vi "winchcontrol2014_TTide_Altimeter_Improved_20150213.vi"() -> ()   [LabVIEW 2014]
uses:
  Instance           1 20Saved   winchcontrol .vi
  Instance           2 20Saved   winchcontrol .vi
  Instance           4 20Saved   winchcontrol .vi
  Instance           3 20Saved   winchcontrol .vi
  isPlaying.vi
  Instance           5 20Saved   winchcontrol .vi
  Instance           6 20Saved   winchcontrol .vi
panel:
  in  "Going up? \ntry to stop at current depth":bool
  out "Too late":string="Too late now!!!  Just pray!"
  out "Current Range":dbl
  out "Fake altimeter yaxis":T1(graph)
  in  "Auto\ndrop":bool
  in  "Final out speed\n[turns/sec]":dbl=4.0 min=0.0 max=4.0 step=0.1 format="%.1f"
  out "pressure":dbl
  out "Dz/Dt":T1(graph)
  out "Payout History":T1(graph)
  out "Conductivity":T1(graph)
  out "Alti Range":T1(graph)
  in  "Path of Image Capture":path=path "/OPG_Winch_MiniCoreDuo/Users/opg/Sites/FCTD_WINCH/LabView.png"
  in  "Screen Capture":bool
  out "Last update string":string="Updated: 10/29/12 6:37:41 PM"
  in  "Port":i32=4050
  in  "Red Lion IP Address":string="192.168.1.160"
  in  "Beep\non wait?":bool=TRUE
  in  "Drive by \nCTD Data":bool=TRUE
  in  "Max. depth [m]":dbl=330.0 min=0.0 max=2200.0 step=1.0 format="%#_4f"
  out "Time @ max":timestamp=timestamp(3434357554.995505 s since 1904-01-01) format="%<%H:%M:%S>T"
  out "Max payout":dbl=26.1 format="%#4.0f"
  out "Max depth":dbl format="%#4.0f"
  in  "Go Up Now":bool
  in  "Final in speed\n[turns/sec]":dbl=0.7 min=0.0 max=4.0 step=0.1 format="%_2f"
  in  "Slow payout (up)\n[turns]":dbl=7.0 min=0.0 max=1500.0 step=1.0
  out "Final in speed":dbl=0.7 min=0.0 max=4.0 step=0.1 format="%3_2g"
  out "Slow payout (up)":dbl=7.0 min=0.0 max=4.0 step=0.1
  out "CTD Miss Count":dbl
  out "Winch Miss Count":dbl=1.0
  out "Sax Status":u8[](array[numeric])=[1, 1, 0, 0, 5, 0, 1, 1, 0, 0]
  out "Depth":T1(graph)
  out "i value":i32
  out "Concat. string":string="$OPGST,1,2,1243"
  out "CTD data":string="2615984408,1.818078,23.842880,5.097004"
  out "Depth":dbl(slide)=1.8080824462346528 min=0.0 max=1200.0 scale format="%#_4f"
  out "*(type *) &x":i32=38
  out "timestamp":u32=2615984408
  out "Temperature":T1(graph)
  out "Param. String":string="$reqparmx:0019;0000$OPGWPM,10,16,+   6,+ 500, 4.2, 2.0,10000,10000,20000,40000,60000,60000,    0.70,    7,;"
  out "Status String":string="$OPGWST,3,1,+   1.8, 266.9,   0,- 0.01,   0.00,   0,   26307,;"
  out "Sax Status Code":dbl=26307.0 format="%#_8f"
  out "Motor Current":dbl
  out "Motor Payout":dbl=266.9
  out "Sheave Payout":dbl
  out "ATM90 Payout":dbl=1.8
  in  "CTD Data  IP Address":string="192.168.1.158"
  in  "Port":i32=2342
  out "bytes written":i32=62
  out "RL Status Received":bool=TRUE
  out "Accel out":dbl=10000.0
  out "Accel in":dbl=10000.0
  out "Winch Action Status":T2(ring)=enum."HOMING"
  out "Winch Control Mode":u16(ring)=3 items=["STOPPED", "MANUAL JOY", "MANUAL POT", "AUTO", "SEMIAUTO"]
  out "Decel stop in":dbl=60000.0
  out "Decel stop out":dbl=60000.0
  out "Decel in":dbl=40000.0
  out "Decel out":dbl=20000.0
  out "Wire in speed":dbl=2.0
  out "Wire out speed":dbl=4.2
  out "Min payout":dbl=6.0
  out "Max payout":dbl=500.0
  out "Current limit out":dbl=10.0
  out "Current limit in":dbl=16.0
  in  "Drop time [min.]":dbl=8.099999999999985 min=0.0 step=0.1 format="%.1f"
  out "output":string
  in  "Stop Now":bool
  in  "Wire in speed\n[turns/sec]":dbl=2.0 min=0.0 max=5.0 step=0.1 format="%3_2f"
  in  "Decel in":dbl=40000.0
  in  "Decel out":dbl=20000.0
  in  "Stop decel in":dbl=60000.0
  in  "Stop decel out":dbl=60000.0
  in  "Accel  in":dbl=10000.0
  in  "Accel out":dbl=10000.0
  in  "Current limit out\n[Amps]":dbl=10.0 min=0.0 max=20.0 step=0.1 format="%_3f"
  in  "Current limit in\n[Amps]":dbl=16.0 min=0.0 max=19.5 format="%_3f"
  out "input":string="$reqparmx:0019;0000$OPGWPM,10,16,+   6,+ 500, 4.2, 2.0,10000,10000,20000,40000,60000,60000,    0.70,    7,;"
  out "Payout":dbl(slide)=1.8 min=0.0 max=1200.0 step=200.0 scale format="%#1_3f"
  out "Velocity Now":dbl(knob)=-0.01 min=-5.0 max=5.0 step=1.0 scale=-5.0..5.0 scale format="%#_1f"
  in  "Max. payout [turns]":dbl=500.0 min=0.0 max=1640.0 step=1.0 format="%#_4f"
  in  "Min. payout [turns]":dbl=6.0 min=0.0 max=2000.0 step=1.0
  in  "Winch Auto Run":bool=TRUE
  out "Enabled":bool=TRUE
  in  "Vel out Init. [turns/sec]":dbl=4.2 min=0.0 max=8.0 step=0.1 format="%_2f"
  out "Target\nDepth":dbl
  # "OPG  FastCTD LabVIEW CONTROLLER"
  # "Winch Variable Controls"
  # "Winch Variable Status"
  # "Communication Setup"
  # "Communication Data"
  # "FCTD DATA"
  # "RED LION CONTROL"
  # "Screen Capture"
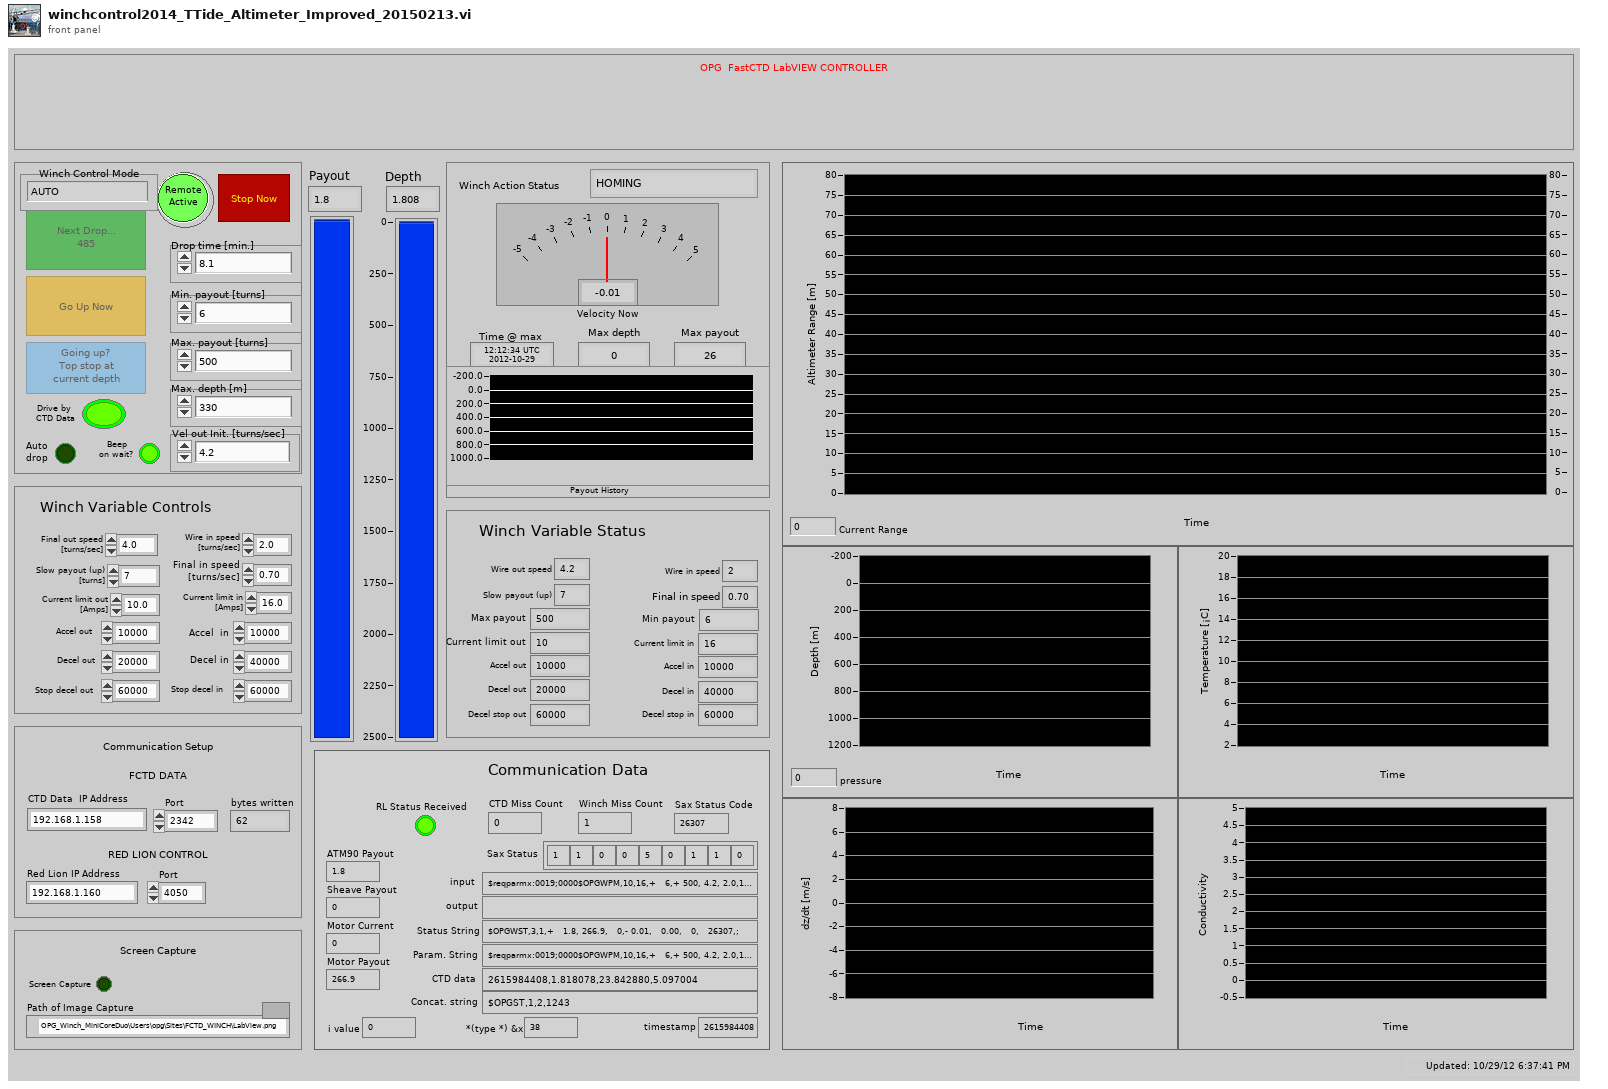
[diagram p1: front panel]
types:
  T1 = cluster{"seconds since 1Jan1904":timestamp, dbl}[]
  T2 = enum16{"START HOMING", "HOMING", "WAIT FOR TRIGGER", "START DROP", "GOING DOWN ?", "GOING UP"}
  T3 = cluster{"Array[0]":dbl, "Array[1]":dbl, "Array[2]":dbl, "Array[3]":dbl, "Array[4]":dbl, "Array[5]":dbl, "Array[6]":dbl, "Array[7]":dbl, "Array[8]":dbl}
  T4 = cluster{"Array[0]":dbl, "Array[1]":dbl, "Array[2]":dbl, "Array[3]":dbl, "Array[4]":dbl, "Array[5]":dbl, "Array[6]":dbl, "Array[7]":dbl, "Array[8]":dbl, "Array[9]":dbl, "Array[10]":dbl, "Array[11]":dbl, "Array[12]":dbl, "Array[13]":dbl}
  T5 = typedef "imagedata.ctl" = cluster{"image type":i32, "image depth":i32, "image":u8[], "mask":u8[], "colors":u32[], "Rectangle":cluster{"left":i16, "top":i16, "right":i16, "bottom":i16}}
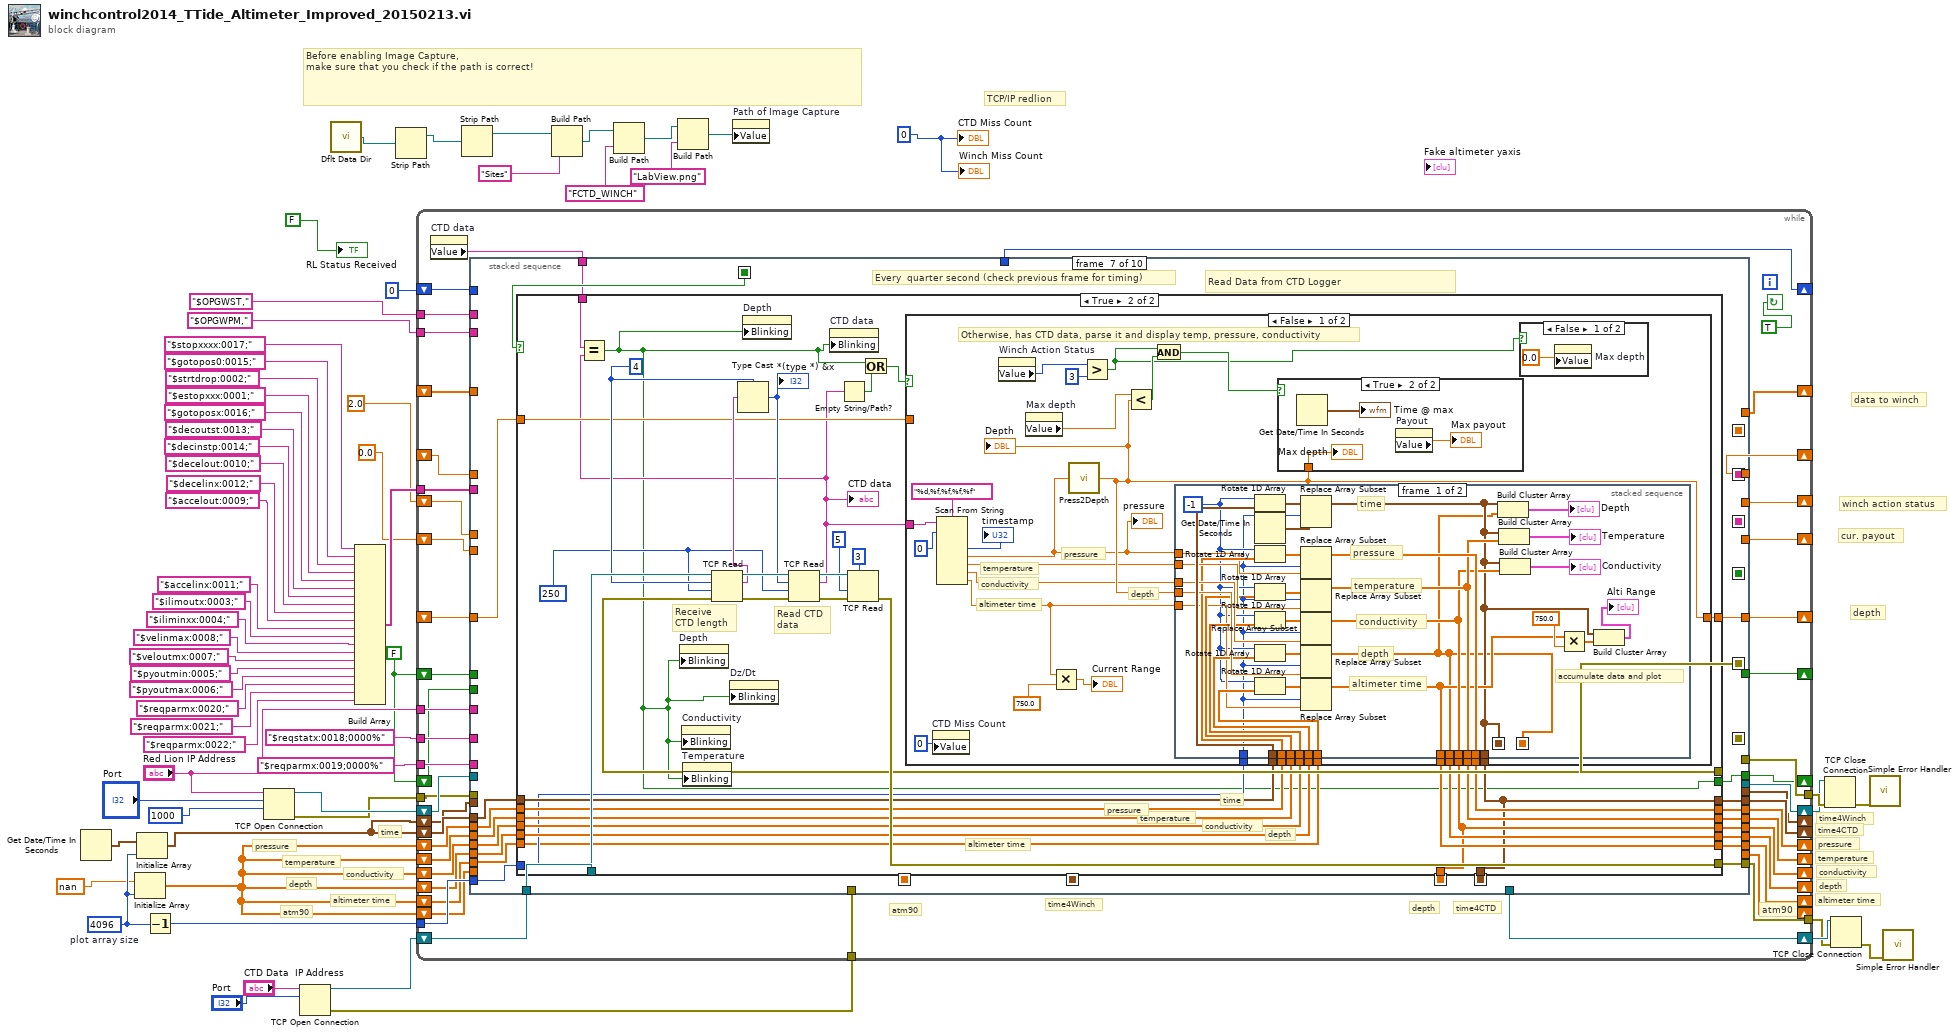
[diagram p0: block diagram]
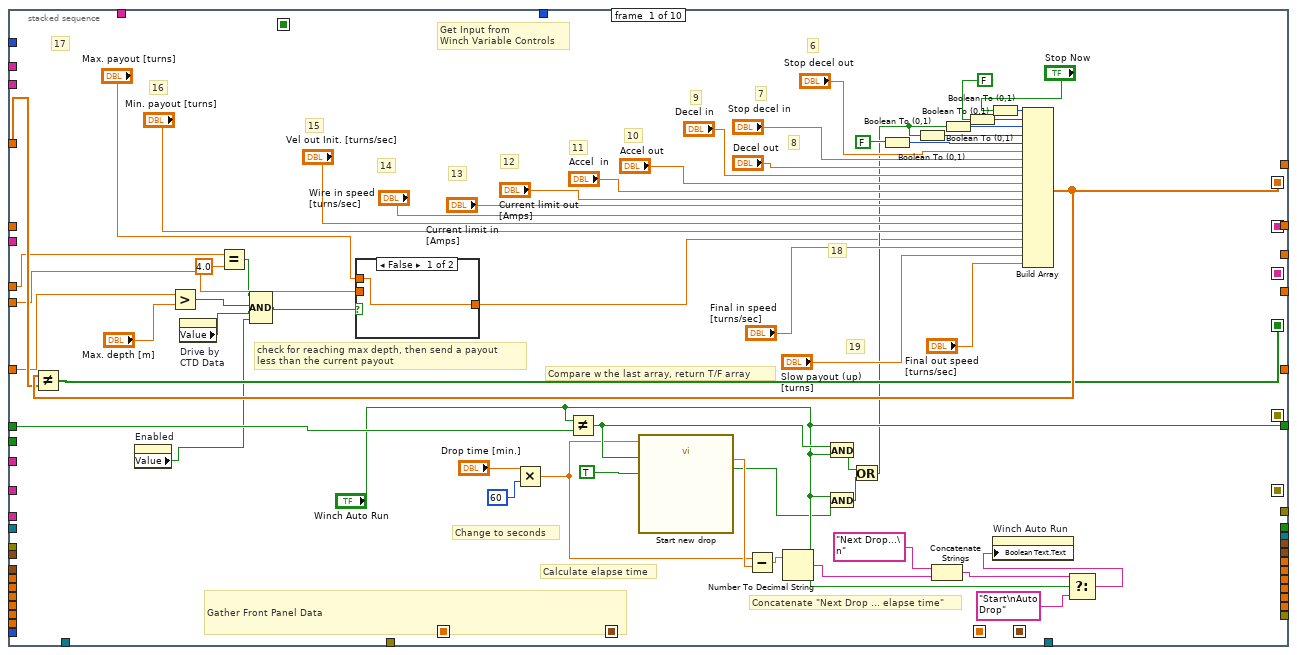
[diagram p2: hidden frame]
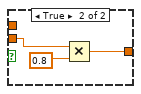
[diagram p3: hidden frame]
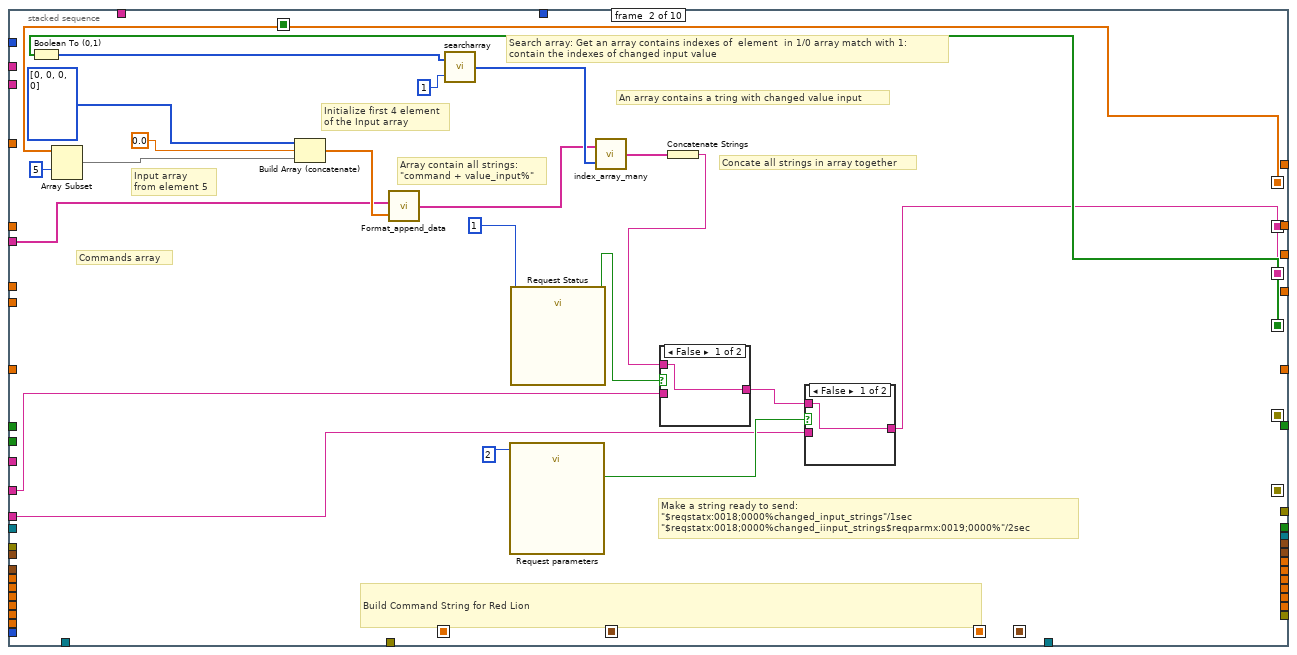
[diagram p4: hidden frame]
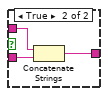
[diagram p5: hidden frame]
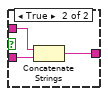
[diagram p6: hidden frame]
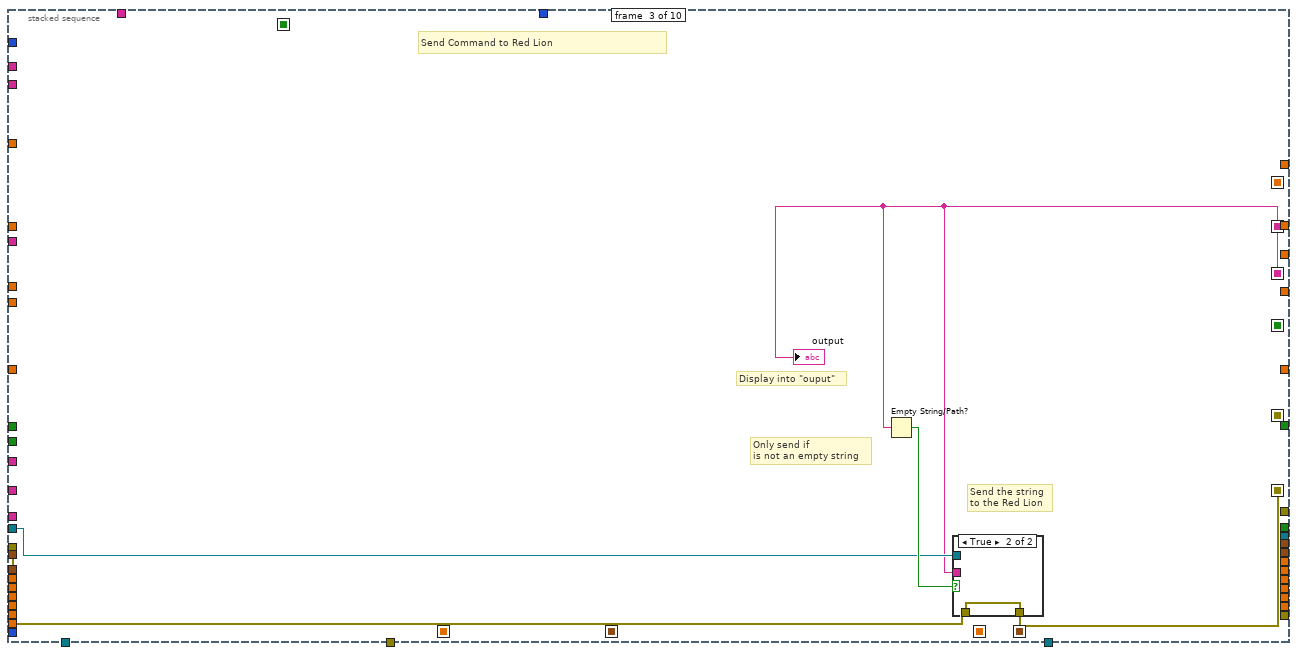
[diagram p7: hidden frame]
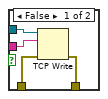
[diagram p8: hidden frame]
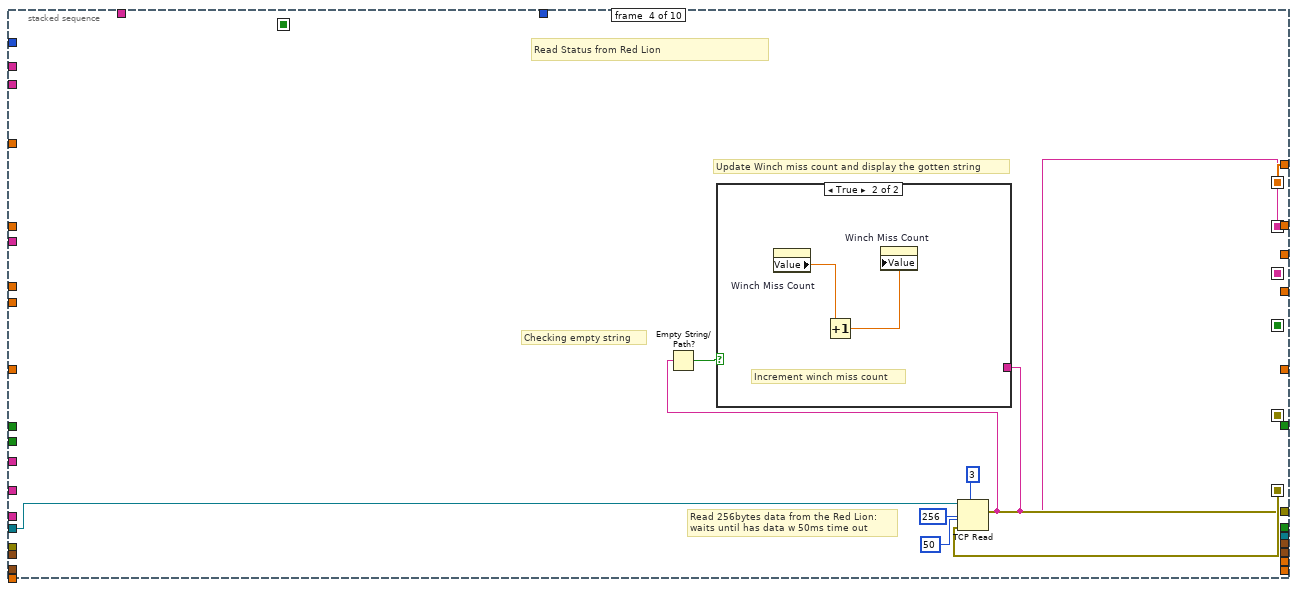
[diagram p9: hidden frame]
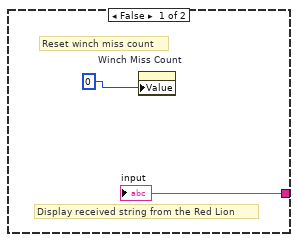
[diagram p10: hidden frame]
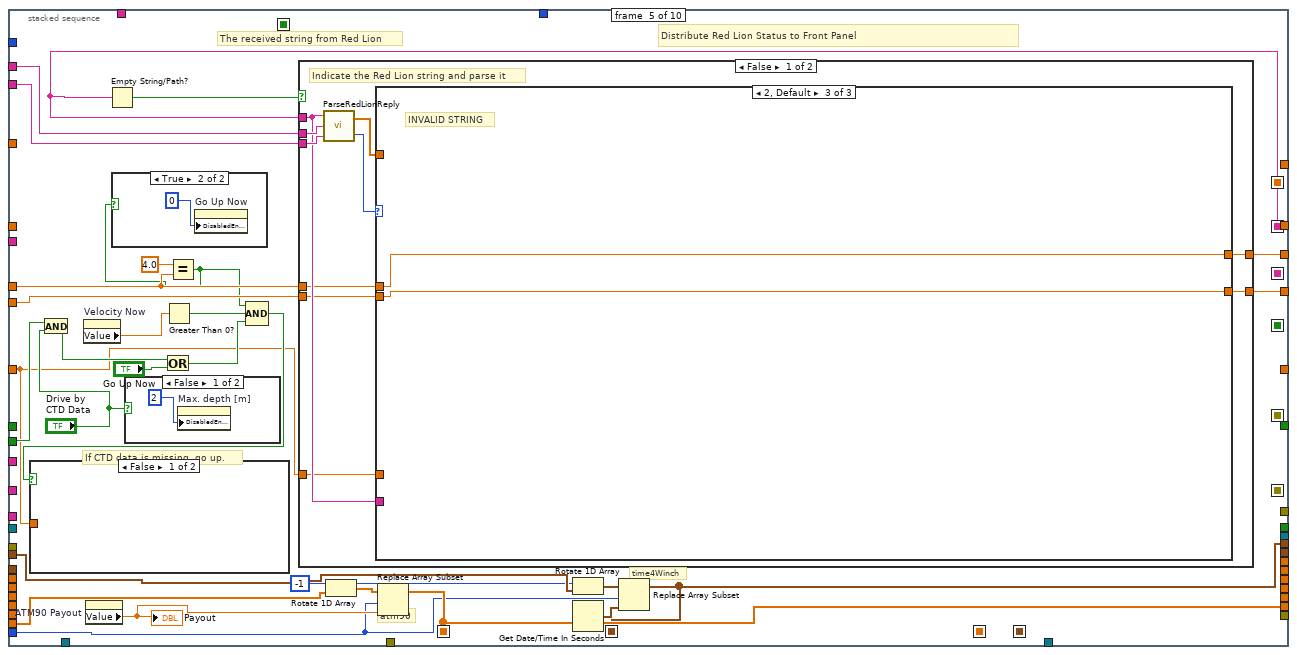
[diagram p11: hidden frame]
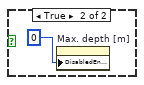
[diagram p12: hidden frame]
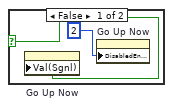
[diagram p13: hidden frame]
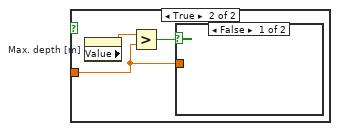
[diagram p14: hidden frame]
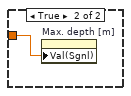
[diagram p15: hidden frame]
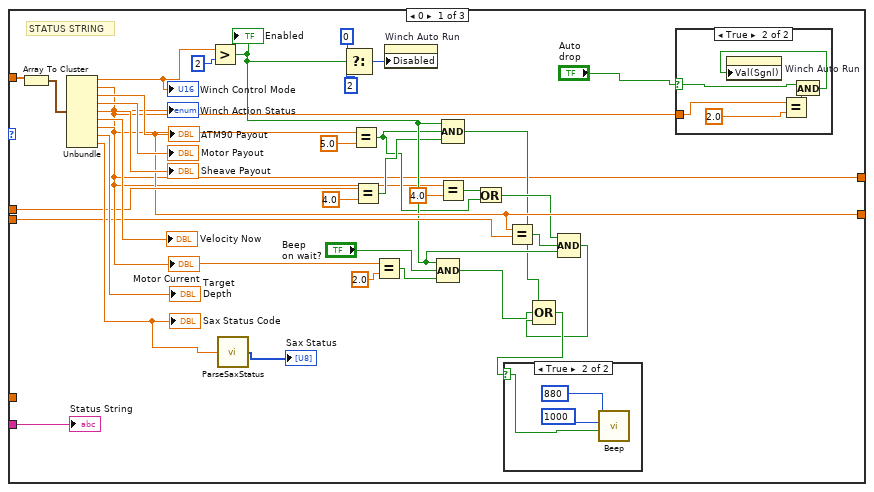
[diagram p16: hidden frame]
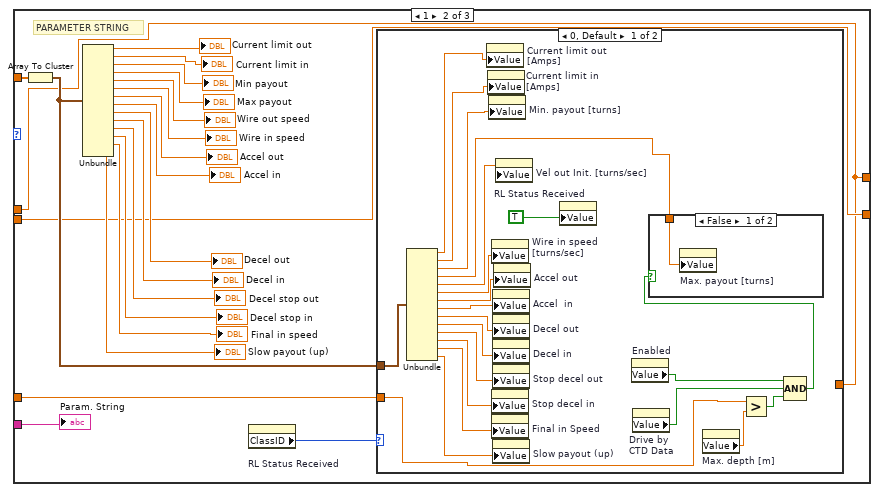
[diagram p19: hidden frame]
diagram:
  w6 = 4096  # plot array size
  w19 = FALSE
  w25 = 0
  # "cur. payout"
  # "depth"
  # "data to winch"
  # "winch action status"
  # "time4Winch"
  # "atm90"
  # "depth"
  # "altimeter time"
  # "altimeter time"
  # "conductivity"
  # "temperature"
  # "time4CTD"
  # "pressure"
  # "depth"
  # "conductivity"
  # "temperature"
  # "time"
  # "pressure"
  # "Before enabling Image Capture, \nmake sure that you check if the path is correct!"
  # "TCP/IP redlion"
  n1 = Get Date/Time In Seconds() -> (seconds since 1Jan1904=w5:timestamp)
  n2 = Initialize Array(nan, w6) -> (w4:dbl[])
  n3 = Initialize Array(w5, w6) -> (w3:timestamp[])
  n4 = Decrement(x=w6) -> (x-1=w7:i32)
  n5 = TCP Open Connection(address="Red Lion IP Address", remote port or service name="Port", timeout ms (60000)=1000) -> (connection ID=w60:refnum<k5>, error out=w58:errorcluster)  [unwired: 2 in]
  n6 = TCP Open Connection(address="CTD Data  IP Address", remote port or service name="Port") -> (connection ID=w34:refnum<k5>, error out=w32:errorcluster)  [unwired: 3 in]
  n7 = call <vilib>:"Dflt Data Dir.vi"() -> ("App:Default Data Directory"=w16:path)
  n8 = Build Array("$stopxxxx:0017;", "$gotopos0:0015;", "$strtdrop:0002;", "$estopxxx:0001;", "$gotoposx:0016;", "$decoutst:0013;", "$decinstp:0014;", "$decelout:0010;", "$decelinx:0012;", "$accelout:0009;", "$accelinx:0011;", "$ilimoutx:0003;", "$iliminxx:0004;", "$velinmax:0008;", "$veloutmx:0007;", "$pyoutmin:0005;", "$pyoutmax:0006;", "$reqparmx:0020;", "$reqparmx:0021;", "$reqparmx:0022;") -> (w56:string[])
  n9 = Strip Path(path=w16) -> (stripped path=w15:path)  [unwired: 1 out]
  n10 = while {
    shift-right: [w110] -> _
    shift-left: _ -> [w108]
    tunnel: w58 -> [w105]
    tunnel: [w109] -> w57
    tunnel: w56 -> [w107]
    tunnel: "$reqstatx:0018;0000%" -> [w104]
    shift-right: [w103] -> _
    shift-left: w19 -> [w102]
    tunnel: w32 -> [w100]
    tunnel: [w99] -> w31
    tunnel: "$reqparmx:0019;0000%" -> [w98]
    shift-right: [w97] -> _
    shift-left: _ -> [w96]
    shift-right: [w95] -> _
    shift-left: 0 -> [w94]
    tunnel: "$OPGWST," -> [w93]
    tunnel: "$OPGWPM," -> [w92]
    shift-right: [w90] -> w24
    shift-left: w60 -> [w106]
    shift-right: [w89] -> w33
    shift-left: w34 -> [w101]
    shift-right: [w88] -> _
    shift-left: _ -> [w87]
    tunnel: "Red Lion IP Address" -> [w85]
    shift-right: [w84] -> _
    shift-left: w19 -> [w83]
    shift-right: [w82] -> _
    shift-left: 2.0 -> [w81]
    shift-right: [w80] -> _
    shift-left: 0.0 -> [w79]
    tunnel: w7 -> [w78]
    shift-right: [w70] -> _
    shift-left: w4 -> [w76]
    shift-right: [w72] -> _
    shift-left: w3 -> [w77]
    shift-right: [w69] -> _
    shift-left: w4 -> [w75]
    shift-right: [w67] -> _
    shift-left: w4 -> [w74]
    shift-right: [w68] -> _
    shift-left: w4 -> [w73]
    shift-right: [w66] -> _
    shift-left: w4 -> [w71]
    shift-right: [w64] -> _
    shift-left: w4 -> [w65]
    shift-right: [w62] -> _
    shift-left: w3 -> [w63]
    stop <- TRUE continue-if-true
    # "time4CTD"
    # "time4Winch"
    # "depth"
    # "atm90"
    # "atm90"
    n11 = property on="CTD data" class="Str"() -> ("Value"=w86:string)  [unwired: 2 in, 2 out]
    n12 = stacked-sequence {
      seq-local: [w165 _ _ _ _ _ _ _ _ _] -> [_ w184 _ w218 _ _ _ _ _ _]
      seq-local: [_ w170 _ _ _ _ _ _ _ _] -> [_ _ w200 _ _ _ _ _ _ _]
      seq-local: [_ _ w201 _ _ _ _ _ _ _] -> [_ _ _ w213 _ _ _ _ _ _]
      seq-local: [w161 _ _ _ _ _ _ _ _ _] -> [_ w191 _ _ _ _ _ _ _ _]
      seq-local: [_ _ _ w211 _ _ _ _ _ _] -> [_ _ _ _ w249 _ _ _ _ _]
      seq-local: [_ _ _ _ _ w369 _ _ _ _] -> [_ _ _ _ _ _ w429 _ _ _]
      seq-local: [_ _ _ _ _ w368 _ _ _ _] -> [_ _ _ _ _ _ w427 _ _ _]
      seq-local: [_ _ _ _ _ _ w409 _ _ _] -> [_ _ _ _ _ _ _ _ _ w662]
      seq-local: [_ _ _ _ w233 _ _ _ _ _] -> [_ _ _ _ _ _ _ _ _ w663]
      seq-local: [_ _ _ _ w228 _ _ _ _ _] -> [_ _ _ _ _ _ _ _ _ w661]
      seq-local: [_ _ _ _ _ _ w408 _ _ _] -> [_ _ _ _ _ _ _ _ _ w660]
      tunnel: w105 -> [_ _ w203 _ _ _ _ _ _ _]
      tunnel: w106 -> [_ _ w202 w214 _ _ _ _ w625 _]
      tunnel: [_ _ _ w218 _ _ _ _ _ _] -> w110
      tunnel: w107 -> [_ w182 _ _ _ _ _ _ _ _]
      tunnel: [_ _ _ w212 _ _ _ _ _ _] -> w109
      tunnel: w108 -> [w164 _ _ _ _ _ _ _ _ _]
      tunnel: w104 -> [_ w176 _ _ _ _ _ _ _ _]
      tunnel: ["Winch Auto Run" _ _ _ _ _ _ _ _ _] -> w103
      tunnel: w102 -> [w141 _ _ _ _ _ _ _ _ _]
      tunnel: w101 -> [_ _ _ _ _ w371 w430 _ w623 _]
      tunnel: w100 -> [_ _ _ _ _ w370 _ _ _ _]
      tunnel: [_ _ _ _ _ _ w428 _ _ _] -> w99
      tunnel: w98 -> [_ w171 _ _ _ _ _ _ _ _]
      tunnel: [_ _ _ _ _ w367 _ _ _ _] -> w97
      tunnel: w96 -> [_ _ _ _ _ w366 _ _ _ _]
      tunnel: w94 -> [_ _ _ _ _ w365 _ _ _ _]
      tunnel: [_ _ _ _ _ w364 _ _ _ _] -> w95
      tunnel: w93 -> [_ _ _ _ w251 _ _ _ _ _]
      tunnel: w92 -> [_ _ _ _ w250 _ _ _ _ _]
      tunnel: [_ _ _ _ _ _ _ _ w624 _] -> w90
      tunnel: [_ _ _ _ _ _ _ _ w622 _] -> w89
      tunnel: [_ _ _ _ _ _ w426 _ _ _] -> w88
      tunnel: w87 -> [w121 _ _ _ w223 _ w425 _ _ _]
      tunnel: w86 -> [_ _ _ _ _ _ w424 _ _ _]
      tunnel: w85 -> [_ _ _ _ _ _ _ _ w621 _]
      tunnel: [_ _ _ _ _ _ w423 _ _ _] -> w84
      tunnel: w83 -> [_ _ _ _ w227 _ _ _ _ _]
      tunnel: [_ _ _ _ w243 _ _ _ _ _] -> w82
      tunnel: w81 -> [w112 _ _ _ w239 _ _ _ _ _]
      tunnel: [_ _ _ _ w242 _ _ _ _ _] -> w80
      tunnel: w79 -> [w118 _ _ _ w241 _ _ _ _ _]
      tunnel: w78 -> [_ _ _ _ w230 _ w422 _ _ _]
      tunnel: w77 -> [_ _ _ _ _ _ w421 _ _ _]
      tunnel: w76 -> [_ _ _ _ _ _ w420 _ _ _]
      tunnel: w75 -> [_ _ _ _ _ _ w419 _ _ _]
      tunnel: w74 -> [_ _ _ _ _ _ w418 _ _ _]
      tunnel: w73 -> [_ _ _ _ _ _ w417 _ _ _]
      tunnel: [_ _ _ _ _ _ w416 _ _ _] -> w72
      tunnel: w71 -> [_ _ _ _ _ _ w415 _ _ _]
      tunnel: [_ _ _ _ _ _ w414 _ _ _] -> w70
      tunnel: [_ _ _ _ _ _ w413 _ _ _] -> w69
      tunnel: [_ _ _ _ _ _ w412 _ _ _] -> w67
      tunnel: [_ _ _ _ _ _ w411 _ _ _] -> w68
      tunnel: [_ _ _ _ _ _ w410 _ _ _] -> w66
      tunnel: w65 -> [_ _ _ _ w237 _ _ _ _ _]
      tunnel: [_ _ _ _ w233 _ _ _ _ _] -> w64
      tunnel: w63 -> [_ _ _ _ w232 _ _ _ _ _]
      tunnel: [_ _ _ _ w228 _ _ _ _ _] -> w62
      frame #0 {
        w162 = FALSE items=["OFF", "ON", "OFF", "ON"] ("Return to top")
        w150 = FALSE items=["OFF", "ON", "OFF", "ON"] ("Go to ...")
        # "check for reaching max depth, then send a payout\nless than the current payout"
        # "19"
        # "18"
        # "17"
        # "16"
        # "15"
        # "14"
        # "13"
        # "12"
        # "11"
        # "10"
        # "9"
        # "8"
        # "7"
        # "6"
        # "Compare w the last array, return T/F array"
        # "Concatenate \"Next Drop ... elapse time\""
        # "Calculate elapse time"
        # "Change to seconds"
        # "Get Input from\nWinch Variable Controls"
        # "Gather Front Panel Data"
        n13 = property on="Enabled" class="Bool (strict)"() -> ("Value"=w115:bool)  [unwired: 2 in, 2 out]
        n14 = Greater?(x=w121, y="Max. depth [m]") -> (0:w117:bool)
        n15 = property on="Drive by \nCTD Data" class="Bool (strict)"() -> ("Value"=w116:bool)  [unwired: 2 in, 2 out]
        n16 = Equal?(x=w112, y=4.0) -> (x = y?=w111:bool)
        n17 = Compound Arithmetic op=AND(w111, w117, w116, w115) -> (w114:bool)
        n18 = case shown="False" w114 {
          tunnel: "Max. payout [turns]" -> [w166 _]
          tunnel: [w166 w168] -> w119
          tunnel: w118 -> [_ w167]
          frame False {
          }
          frame True {
            n19 = Multiply(x=w167, y=0.8) -> (x*y=w168:dbl)
          }
        }
        n20 = Multiply(x="Drop time [min.]", y=60) -> (x*y=w136:dbl)
        n21 = Not Equal?(x="Winch Auto Run", y=w141) -> (x != y?=w140:bool)
        n22 = call "Start new drop"("Time Target (s)"=w136, "Reset"=w140, "Auto Reset"=TRUE) -> ("Elapsed Time (s)"=w137:dbl, "Time has Elapsed"=w126:bool)  [unwired: 9 in, 6 out]
        n23 = Subtract(x=w136, y=w137) -> (x-y=w135:dbl)
        n24 = Number To Decimal String(number=w135) -> (decimal integer string=w134:string)  [unwired: 1 in]
        n25 = And(x=w140, y="Winch Auto Run") -> (x .and. y?=w139:bool)
        n26 = And(x="Winch Auto Run", y=w126) -> (x .and. y?=w138:bool)
        n27 = Or(x=w139, y=w138) -> (x .or. y?=w124:bool)
        n28 = Boolean To (0,1)(Boolean=w150) -> (0, 1=w149:i16)
        n29 = Boolean To (0,1)(Boolean=w124) -> (0, 1=w148:i16)
        n30 = Concatenate Strings("Next Drop...\n", w134) -> (w131:string)
        n31 = Boolean To (0,1)(Boolean=w124) -> (0, 1=w147:i16)
        n32 = Boolean To (0,1)(Boolean=w162) -> (0, 1=w146:i16)
        n33 = Boolean To (0,1)(Boolean="Stop Now") -> (0, 1=w145:i16)
        n34 = Build Array(w145, w146, w147, w148, w149, "Stop decel out", "Stop decel in", "Decel out", "Decel in", "Accel out", "Accel  in", "Current limit out\n[Amps]", "Current limit in\n[Amps]", "Wire in speed\n[turns/sec]", "Vel out Init. [turns/sec]", "Min. payout [turns]", w119, "Final in speed\n[turns/sec]", "Slow payout (up)\n[turns]", "Final out speed\n[turns/sec]") -> (w165:dbl[])
        n35 = Not Equal?(x=w165, y=w164) -> (x != y?=w161:bool[])
        n36 = Select(t=w131, s="Winch Auto Run", f="Start\nAuto Drop") -> (s? t:f=w132:string)
        n37 = property on="Winch Auto Run" class="Bool (strict)"("Boolean Text.Text"=w132) -> ()  [unwired: 2 in, 2 out]
      }
      frame #1 {
        # "Make a string ready to send:\n\"$reqstatx:0018;0000%changed_input_strings\"/1sec\n\"$reqstatx:0018;0000%changed_iinput_strings$reqparmx:0019;0000%\"/2sec"
        # "Concate all strings in array together"
        # "An array contains a tring with changed value input"
        # "Array contain all strings:\n\"command + value_input%\""
        # "Commands array"
        # "Initialize first 4 element\nof the Input array"
        # "Input array\nfrom element 5"
        # "Search array: Get an array contains indexes of  element  in 1/0 array match with 1:\ncontain the indexes of changed input value"
        # "Build Command String for Red Lion"
        n38 = Boolean To (0,1)(Boolean=w191) -> (0, 1=w189:i16[])
        n39 = Array Subset(array=w184, index=5) -> (w180:dbl[])  [unwired: 1 in]
        n40 = Build Array (concatenate)(i32[] [0, 0, 0, 0], 0.0 ("Depth to go to"), w180) -> (w183:dbl[])
        n41 = call "Format_append_data.vi"("Numbers to append"=w183, "Strings without numbers"=w182) -> ("Final Strings"=w181:string[])
        n42 = call "searcharray.vi"("Search character"=1, "Array 2"=w189) -> ("Array"=w188:i16[])
        n43 = call "Request parameters"("Time Target (s)"=2) -> ("Time has Elapsed"=w172:bool)  [unwired: 11 in, 7 out]
        n44 = call "Request Status"("Time Target (s)"=1) -> ("Time has Elapsed"=w177:bool)  [unwired: 11 in, 7 out]
        n45 = call "index_array_many.vi"("Lines of Array to grab"=w188, "String Array Input"=w181) -> ("Output array"=w187:string[])
        n46 = Concatenate Strings(w187) -> (w175:string)
        n47 = case shown="False" w177 {
          tunnel: w175 -> [w196 w199]
          tunnel: [w196 w198] -> w173
          tunnel: w176 -> [_ w197]
          frame False {
          }
          frame True {
            n48 = Concatenate Strings(w199, w197) -> (w198:string)
          }
        }
        n49 = case shown="False" w172 {
          tunnel: w173 -> [w192 w195]
          tunnel: [w192 w194] -> w170
          tunnel: w171 -> [_ w193]
          frame False {
          }
          frame True {
            n50 = Concatenate Strings(w195, w193) -> (w194:string)
          }
        }
      }
      frame #2 {
        # "Send the string\nto the Red Lion"
        # "Only send if\nis not an empty string"
        # "Display into \"ouput\""
        # "Send Command to Red Lion"
        n51 = Empty String/Path?(string/path=w200) -> (empty?=w204:bool)
        n52 = case shown="True" w204 {
          tunnel: w200 -> [w207 _]
          tunnel: w202 -> [w208 _]
          tunnel: w203 -> [w206 w209]
          tunnel: [w205 w209] -> w201
          frame False {
            n53 = TCP Write(connection ID=w208, data in=w207, error in (no error)=w206) -> (error out=w205:errorcluster)  [unwired: 1 in, 2 out]
          }
          frame True {
          }
        }
        "output" <- w200
      }
      frame #3 {
        # "Update Winch miss count and display the gotten string"
        # "Checking empty string"
        # "Read 256bytes data from the Red Lion:\nwaits until has data w 50ms time out"
        # "Read Status from Red Lion"
        n54 = TCP Read(connection ID=w214, bytes to read=256, error in (no error)=w213, 7:3, 9:50) -> (data out=w211:string, error out=w212:errorcluster)  [unwired: 1 out]
        n55 = Empty String/Path?(string/path=w211) -> (empty?=w210:bool)
        n56 = case shown="True" w210 {
          tunnel: w211 -> [w220 _]
          frame False {
            # "Display received string from the Red Lion"
            # "Reset winch miss count"
            n57 = property on="Winch Miss Count" class="DigNum (strict)"("Value"=0) -> ()  [unwired: 2 in, 2 out]
            "input" <- w220
          }
          frame True {
            # "Increment winch miss count"
            n58 = property on="Winch Miss Count" class="DigNum (strict)"() -> ("Value"=w222:dbl)  [unwired: 2 in, 2 out]
            n59 = Increment(x=w222) -> (x+1=w221:dbl)
            n60 = property on="Winch Miss Count" class="DigNum (strict)"("Value"=w221) -> ()  [unwired: 2 in, 2 out]
          }
        }
      }
      frame #4 {
        w231 = -1
        # "If CTD data is missing, go up."
        # "time4Winch"
        # "atm90"
        # "The received string from Red Lion"
        # "Distribute Red Lion Status to Front Panel"
        n61 = And(x=w227, y="Drive by \nCTD Data") -> (x .and. y?=w226:bool)
        n62 = property on="Velocity Now" class="Knob (strict)"() -> ("Value"=w247:dbl)  [unwired: 2 in, 2 out]
        n63 = property on="ATM90 Payout" class="DigNum (strict)"() -> ("Value"=w235:dbl)  [unwired: 2 in, 2 out]
        "Payout" <- w235
        n64 = Empty String/Path?(string/path=w249) -> (empty?=w248:bool)
        n65 = case shown="False" "Drive by \nCTD Data" {
          frame False {
            n66 = property on="Max. depth [m]" class="DigNum (strict)"("DisabledEnum"=2) -> ()  [unwired: 2 in, 2 out]
          }
          frame True {
            n67 = property on="Max. depth [m]" class="DigNum (strict)"("DisabledEnum"=0) -> ()  [unwired: 2 in, 2 out]
          }
        }
        n68 = Or(x=w226, y="Go Up Now") -> (x .or. y?=w244:bool)
        n69 = Greater Than 0?(x=w247) -> (x > 0?=w245:bool)
        n70 = Equal?(x=4.0, y=w239) -> (x = y?=w238:bool)
        n71 = case shown="True" w238 {
          selector: w238 -> [w254 _]
          frame False {
            n72 = property on="Go Up Now" class="Bool (strict)"("Val(Sgnl)"=w254) -> ()  [unwired: 2 in, 2 out]
            n73 = property on="Go Up Now" class="Bool (strict)"("DisabledEnum"=2) -> ()  [unwired: 2 in, 2 out]
          }
          frame True {
            n74 = property on="Go Up Now" class="Bool (strict)"("DisabledEnum"=0) -> ()  [unwired: 2 in, 2 out]
          }
        }
        n75 = Compound Arithmetic op=AND(w238, w245, w244) -> (w246:bool)
        n76 = case shown="False" w246 {
          tunnel: w223 -> [_ w257]
          frame False {
          }
          frame True {
            n77 = property on="Max. depth [m]" class="DigNum (strict)"() -> ("Value"=w259:dbl)  [unwired: 2 in, 2 out]
            n78 = Greater?(x=w259, y=w257) -> (0:w258:bool)
            n79 = case shown="False" w258 {
              tunnel: w257 -> [_ w260]
              frame False {
              }
              frame True {
                n80 = property on="Max. depth [m]" class="DigNum (strict)"("Val(Sgnl)"=w260) -> ()  [unwired: 2 in, 2 out]
              }
            }
          }
        }
        n81 = case shown="False" w248 {
          tunnel: w251 -> [w268 _]
          tunnel: w250 -> [w267 _]
          tunnel: w249 -> [w266 _]
          tunnel: [w265 w362] -> w243
          tunnel: w239 -> [w264 w362]
          tunnel: [w263 w361] -> w242
          tunnel: w241 -> [w262 w361]
          tunnel: w223 -> [w261 _]
          frame False {
            # "Indicate the Red Lion string and parse it"
            n82 = call "ParseRedLionReply.vi"("Parameter Iidicator"=w267, "Status Indicator"=w268, "Red Lion String"=w266) -> ("Type"=w270:i16, "Array"=w269:dbl[])
            n83 = case shown="2, Default" w270 {
              tunnel: w269 -> [w305 w335 _]
              tunnel: w266 -> [w297 w321 _]
              tunnel: [w272 w316 w360] -> w265
              tunnel: w264 -> [w288 w316 w360]
              tunnel: [w287 w318 w359] -> w263
              tunnel: w262 -> [w286 w318 w359]
              tunnel: w261 -> [_ w315 _]
              frame 0 {
                # "STATUS STRING"
                n84 = Array To Cluster(array=w305) -> (cluster=w304:T3)
                n85 = Unbundle(w304) -> ("Array[0]"=w303:dbl, "Array[1]"=w272:dbl, "Array[2]"=w287:dbl, "Array[3]"=→"Motor Payout":dbl, "Array[4]"=→"Sheave Payout":dbl, "Array[5]"=→"Velocity Now":dbl, "Array[6]"=→"Motor Current":dbl, "Array[7]"=→"Target\nDepth":dbl, "Array[8]"=w293:dbl)
                "Winch Control Mode" <- w303
                "Winch Action Status" <- w272
                "ATM90 Payout" <- w287
                "Sax Status Code" <- w293
                n86 = Greater?(x=w303, y=2) -> (0:w281:bool)
                "Enabled" <- w281
                n87 = call "ParseSaxStatus.vi"("Status Code In"=w293) -> ("Status Flags"=→"Sax Status":i8[])
                n88 = Select(t=0, s=w281, f=2) -> (s? t:f=w294:i32)
                n89 = Equal?(x=w272, y=5.0) -> (x = y?=w274:bool)
                n90 = Equal?(x=w288, y=4.0) -> (x = y?=w278:bool)
                n91 = Equal?(x=w272, y=2.0) -> (x = y?=w280:bool)
                n92 = property on="Winch Auto Run" class="Bool (strict)"("Disabled"=w294) -> ()  [unwired: 2 in, 2 out]
                n93 = Compound Arithmetic op=AND(w281, "Beep\non wait?", w280) -> (w275:bool)
                n94 = Equal?(x=w272, y=4.0) -> (x = y?=w284:bool)
                n95 = Compound Arithmetic op=AND(w281, w274, w278) -> (w277:bool)
                n96 = Or(x=w284, y=w274) -> (x .or. y?=w283:bool)
                n97 = Equal?(x=w287, y=w286) -> (x = y?=w282:bool)
                n98 = Compound Arithmetic op=AND(w283, w282, w281) -> (w273:bool)
                n99 = Compound Arithmetic op=OR(w277, w275, w273) -> (w276:bool)
                n100 = case shown="True" w276 {
                  selector: w276 -> [_ w312]
                  frame False {
                  }
                  frame True {
                    n101 = call <vilib>:"Beep.vi"("use system alert? (T) - ignored"=w312, "duration (msec) - ignored"=u32 1000, "frequency (Hz) - ignored"=u32 880) -> ()  [unwired: 9 in]
                  }
                }
                n102 = case shown="True" "Auto\ndrop" {
                  selector: "Auto\ndrop" -> [_ w308]
                  tunnel: w272 -> [_ w310]
                  frame False {
                  }
                  frame True {
                    n103 = Equal?(x=w310, y=2.0) -> (x = y?=w309:bool)
                    n104 = And(x=w308, y=w309) -> (x .and. y?=w307:bool)
                    n105 = property on="Winch Auto Run" class="Bool (strict)"("Val(Sgnl)"=w307) -> ()  [unwired: 2 in, 2 out]
                  }
                }
                "Status String" <- w297
              }
              frame 1 {
                # "PARAMETER STRING"
                n106 = Array To Cluster(array=w335) -> (cluster=w322:T4)
                n107 = Unbundle(w322) -> ("Array[0]"=→"Current limit out":dbl, "Array[1]"=→"Current limit in":dbl, "Array[2]"=→"Min payout":dbl, "Array[3]"=→"Max payout":dbl, "Array[4]"=→"Wire out speed":dbl, "Array[5]"=→"Wire in speed":dbl, "Array[6]"=→"Accel out":dbl, "Array[7]"=→"Accel in":dbl, "Array[8]"=→"Decel out":dbl, "Array[9]"=→"Decel in":dbl, "Array[10]"=→"Decel stop out":dbl, "Array[11]"=→"Decel stop in":dbl, "Array[12]"=→"Final in speed":dbl, "Array[13]"=→"Slow payout (up)":dbl)
                n108 = property on="RL Status Received" class="Bool (strict)"() -> ("ClassID"=w317:u32)  [unwired: 2 in, 2 out]
                n109 = case shown="0, Default" w317 {
                  tunnel: w322 -> [w357 _]
                  tunnel: w316 -> [_ _]
                  tunnel: w315 -> [w341 _]
                  frame 0, Default {
                    n110 = Unbundle(w357) -> ("Array[0]"=w356:dbl, "Array[1]"=w355:dbl, "Array[2]"=w354:dbl, "Array[3]"=w342:dbl, "Array[4]"=w353:dbl, "Array[5]"=w352:dbl, "Array[6]"=w346:dbl, "Array[7]"=w351:dbl, "Array[8]"=w350:dbl, "Array[9]"=w349:dbl, "Array[10]"=w348:dbl, "Array[11]"=w347:dbl, "Array[12]"=w345:dbl, "Array[13]"=w344:dbl)
                    n111 = property on="Current limit out\n[Amps]" class="DigNum (strict)"("Value"=w356) -> ()  [unwired: 2 in, 2 out]
                    n112 = property on="Current limit in\n[Amps]" class="DigNum (strict)"("Value"=w355) -> ()  [unwired: 2 in, 2 out]
                    n113 = property on="Min. payout [turns]" class="DigNum (strict)"("Value"=w354) -> ()  [unwired: 2 in, 2 out]
                    n114 = property on="Wire in speed\n[turns/sec]" class="DigNum (strict)"("Value"=w352) -> ()  [unwired: 2 in, 2 out]
                    n115 = property on="Stop decel in" class="DigNum (strict)"("Value"=w347) -> ()  [unwired: 2 in, 2 out]
                    n116 = property on="Final in Speed" class="DigNum (strict)"("Value"=w345) -> ()  [unwired: 2 in, 2 out]
                    n117 = property on="Accel  in" class="DigNum (strict)"("Value"=w351) -> ()  [unwired: 2 in, 2 out]
                    n118 = property on="Decel out" class="DigNum (strict)"("Value"=w350) -> ()  [unwired: 2 in, 2 out]
                    n119 = property on="Decel in" class="DigNum (strict)"("Value"=w349) -> ()  [unwired: 2 in, 2 out]
                    n120 = property on="Stop decel out" class="DigNum (strict)"("Value"=w348) -> ()  [unwired: 2 in, 2 out]
                    n121 = property on="Slow payout (up)" class="DigNum (strict)"("Value"=w344) -> ()  [unwired: 2 in, 2 out]
                    n122 = property on="Accel out" class="DigNum (strict)"("Value"=w346) -> ()  [unwired: 2 in, 2 out]
                    n123 = property on="Vel out Init. [turns/sec]" class="DigNum (strict)"("Value"=w353) -> ()  [unwired: 2 in, 2 out]
                    n124 = property on="RL Status Received" class="Bool (strict)"("Value"=TRUE) -> ()  [unwired: 2 in, 2 out]
                    n125 = property on="Enabled" class="Bool (strict)"() -> ("Value"=w339:bool)  [unwired: 2 in, 2 out]
                    n126 = property on="Drive by \nCTD Data" class="Bool (strict)"() -> ("Value"=w338:bool)  [unwired: 2 in, 2 out]
                    n127 = property on="Max. depth [m]" class="DigNum (strict)"() -> ("Value"=w340:dbl)  [unwired: 2 in, 2 out]
                    n128 = Greater?(x=w341, y=w340) -> (0:w337:bool)
                    n129 = Compound Arithmetic op=AND(w339, w338, w337) -> (w336:bool)
                    n130 = case shown="False" w336 {
                      tunnel: w342 -> [w358 _]
                      frame False {
                        n131 = property on="Max. payout [turns]" class="DigNum (strict)"("Value"=w358) -> ()  [unwired: 2 in, 2 out]
                      }
                      frame True {
                      }
                    }
                  }
                  frame 1 {
                  }
                }
                "Param. String" <- w321
              }
              frame 2, Default {
                # "INVALID STRING"
              }
            }
          }
          frame True {
            # "If empty string, do nothing"
          }
        }
        n132 = Rotate 1D Array(1:w237, 2:w231) -> (0:w236:dbl[])
        n133 = Replace Array Subset(array=w236, new element=w235, index=w230) -> (w233:dbl[])
        n134 = Rotate 1D Array(1:w232, 2:w231) -> (0:w234:timestamp[])
        n135 = Get Date/Time In Seconds() -> (seconds since 1Jan1904=w229:timestamp)
        n136 = Replace Array Subset(array=w234, new element=w229, index=w230) -> (w228:timestamp[])
      }
      frame #5 {
        # "Time between\n each\nrequest for \nCTD data"
        # "Send Status to CTD Logger"
        n137 = call "Send to FastCTD  logger"("Time Target (s)"=0.25) -> ("Time has Elapsed"=w368:bool)  [unwired: 11 in, 7 out]
        n138 = case shown="True" w368 {
          tunnel: w371 -> [_ w384]
          tunnel: w370 -> [w374 w383]
          tunnel: [w374 w382] -> w369
          tunnel: [w373 w378] -> w367
          tunnel: w366 -> [w373 w377]
          tunnel: w365 -> [w372 w376]
          tunnel: [w372 w375] -> w364
          frame False {
          }
          frame True {
            n139 = property on="Status String" class="Str"() -> ("Value"=w380:string)  [unwired: 2 in, 2 out]
            n140 = Empty String/Path?(string/path=w380) -> (empty?=w381:bool)
            n141 = case shown="True" w381 {
              tunnel: w380 -> [w388 _]
              tunnel: [w388 w398] -> w379
              tunnel: [w387 w392] -> w378
              tunnel: w377 -> [w387 w391]
              tunnel: w376 -> [w386 w390]
              tunnel: [w386 w389] -> w375
              frame False {
              }
              frame True {
                # "Since Status string is empty, make a string \"$OPGST,1,2/3,1243\"\nto send to FCTD app"
                n142 = Increment(x=w390) -> (x+1=w389:i32)
                n143 = Quotient & Remainder(x=w389, y=4) -> (x-y*floor(x/y)=w395:i32)  [unwired: 1 out]
                n144 = Equal To 0?(x=w395) -> (x = 0?=w394:bool)
                n145 = case shown="True" w394 {
                  tunnel: [w401 w403] -> w393
                  tunnel: [w401 w403] -> w392
                  tunnel: w391 -> [w401 w402]
                  frame False {
                  }
                  frame True {
                    n146 = Equal?(x=w402, y=3.0) -> (x = y?=w404:bool)
                    n147 = Select(t=2.0 ("y"), s=w404, f=3.0 ("y")) -> (s? t:f=w403:dbl)
                  }
                }
                n148 = Number To Decimal String(number=w393) -> (decimal integer string=w397:string)  [unwired: 1 in]
                n149 = Concatenate Strings("$OPGST,1," ("string"), w397, ",1243" ("string")) -> (w398:string)
                "Concat. string" <- w398
              }
            }
            n150 = TCP Write(connection ID=w384, data in=w379, error in (no error)=w383) -> (bytes written=→"bytes written":i32, error out=w382:errorcluster)  [unwired: 1 in, 1 out]
          }
        }
        "i value" <- w365
      }
      frame #6 {
        # "Every  quarter second (check previous frame for timing)"
        # "Read Data from CTD Logger"
        n151 = case shown="True" w427 {
          selector: w427 -> [w437 _]
          tunnel: w430 -> [_ w472]
          tunnel: w429 -> [w439 w457]
          tunnel: [w439 w465] -> w428
          tunnel: [w438 w461] -> w426
          tunnel: w425 -> [w438 w460]
          tunnel: w424 -> [_ w458]
          tunnel: [w437 w442] -> w423
          tunnel: w422 -> [_ w450]
          tunnel: w421 -> [w432 w455]
          tunnel: w420 -> [w436 w454]
          tunnel: w419 -> [w435 w453]
          tunnel: w418 -> [w434 w452]
          tunnel: w417 -> [w431 w451]
          tunnel: [w432 w443] -> w416
          tunnel: w415 -> [w433 w449]
          tunnel: [w436 w448] -> w414
          tunnel: [w435 w447] -> w413
          tunnel: [w434 w444] -> w412
          tunnel: [w431 w446] -> w411
          tunnel: [w433 w445] -> w410
          tunnel: [w431 w444] -> w409
          tunnel: [w432 w443] -> w408
          frame False {
          }
          frame True {
            w456 = 250
            w471 = 4
            # "altimeter time"
            # "depth"
            # "conductivity"
            # "temperature"
            # "time"
            # "pressure"
            # "Read CTD\ndata"
            # "Receive\nCTD length"
            n152 = TCP Read(connection ID=w472, bytes to read=w471, error in (no error)=w457, 9:w456) -> (connection ID out=w470:refnum<k5>, data out=w469:string, error out=w467:errorcluster)  [unwired: 1 in]
            n153 = Type Cast(type=w471, x=w469) -> (*(type *) &x=w468:i32)
            "*(type *) &x" <- w468
            n154 = TCP Read(connection ID=w470, bytes to read=w468, error in (no error)=w467, 9:w456) -> (connection ID out=w464:refnum<k5>, data out=w459:string, error out=w466:errorcluster)  [unwired: 1 in]
            "CTD data" <- w459
            n155 = Equal?(x=w458, y=w459) -> (x = y?=w442:bool)
            n156 = property on="Depth" class="XYGraph (strict)"("Blinking"=w442) -> ()  [unwired: 2 in, 2 out]
            n157 = property on="Conductivity" class="XYGraph (strict)"("Blinking"=w442) -> ()  [unwired: 2 in, 2 out]
            n158 = property on="Temperature" class="XYGraph (strict)"("Blinking"=w442) -> ()  [unwired: 2 in, 2 out]
            n159 = property on="Dz/Dt" class="XYGraph (strict)"("Blinking"=w442) -> ()  [unwired: 2 in, 2 out]
            n160 = property on="Depth" class="Slide (strict)"("Blinking"=w442) -> ()  [unwired: 2 in, 2 out]
            n161 = property on="CTD data" class="Str"("Blinking"=w442) -> ()  [unwired: 2 in, 2 out]
            n162 = Empty String/Path?(string/path=w459) -> (empty?=w441:bool)
            n163 = TCP Read(connection ID=w464, error in (no error)=w466, 7:3, 9:5) -> (error out=w465:errorcluster)  [unwired: 1 in, 2 out]
            n164 = Or(x=w442, y=w441) -> (x .or. y?=w440:bool)
            n165 = case shown="False" w440 {
              tunnel: w459 -> [w500 _]
              tunnel: [w492 w570] -> w461
              tunnel: w460 -> [_ w570]
              tunnel: w455 -> [w491 w567]
              tunnel: w454 -> [w490 w566]
              tunnel: w453 -> [w489 w565]
              tunnel: w452 -> [w488 w564]
              tunnel: w451 -> [w487 w563]
              tunnel: w450 -> [w486 _]
              tunnel: [w485 w567] -> w443
              tunnel: w449 -> [w484 w562]
              tunnel: [w483 w566] -> w448
              tunnel: [w481 w565] -> w447
              tunnel: [w479 w564] -> w444
              tunnel: [w478 w563] -> w446
              tunnel: [w477 w562] -> w445
              frame False {
                # "depth"
                # "altimeter time"
                # "conductivity"
                # "temperature"
                # "pressure"
                # "Otherwise, has CTD data, parse it and display temp, pressure, conductivity"
                n166 = property on="CTD Miss Count" class="DigNum (strict)"("Value"=0) -> ()  [unwired: 2 in, 2 out]
                n167 = Scan From String(format string="%d,%f,%f,%f,%f", input string=w500, initial scan location=u32 0) -> (output 1=→"timestamp":u32, output 2=w473:dbl, output 3=w482:dbl, output 4=w480:dbl, output 5=w474:dbl)  [unwired: 6 in, 3 out]
                "pressure" <- w473
                n168 = property on="Winch Action Status" class="Enum (strict)"() -> ("Value"=w499:T2)  [unwired: 2 in, 2 out]
                n169 = property on="Max depth" class="DigNum (strict)"() -> ("Value"=w497:dbl)  [unwired: 2 in, 2 out]
                n170 = Multiply(x=w474, y=750.0) -> (x*y=→"Current Range":dbl)
                n171 = call "Press2Depth.vi"("Pressure in dbars"=w473) -> ("Depth in meters"=w492:dbl)
                "Depth" <- w492
                n172 = Greater?(x=w499, y=3) -> (0:w494:bool)
                n173 = Less?(x=w497, y=w492) -> (x < y?=w496:bool)
                n174 = And(x=w494, y=w496) -> (x .and. y?=w495:bool)
                n175 = stacked-sequence {
                  seq-local: [w505 _] -> [_ w540]
                  seq-local: [w507 _] -> [_ w539]
                  tunnel: w492 -> [w528 _]
                  tunnel: w491 -> [w536 _]
                  tunnel: w490 -> [w525 _]
                  tunnel: w489 -> [w526 _]
                  tunnel: w488 -> [w527 _]
                  tunnel: w487 -> [w524 _]
                  tunnel: w486 -> [w511 _]
                  tunnel: [w507 _] -> w485
                  tunnel: w484 -> [w521 _]
                  tunnel: w473 -> [w523 _]
                  tunnel: [w517 _] -> w483
                  tunnel: w482 -> [w531 _]
                  tunnel: [w515 _] -> w481
                  tunnel: w480 -> [w529 _]
                  tunnel: w474 -> [w519 _]
                  tunnel: [w512 _] -> w479
                  tunnel: [w505 _] -> w478
                  tunnel: [w509 _] -> w477
                  frame #0 {
                    w518 = -1
                    # "accumulate data and plot"
                    # "depth"
                    # "altimeter time"
                    # "conductivity"
                    # "temperature"
                    # "time"
                    # "pressure"
                    n176 = Rotate 1D Array(1:w536, 2:w518) -> (0:w535:timestamp[])
                    n177 = Get Date/Time In Seconds() -> (seconds since 1Jan1904=w534:timestamp)
                    n178 = Rotate 1D Array(1:w525, 2:w518) -> (0:w533:dbl[])
                    n179 = Rotate 1D Array(1:w526, 2:w518) -> (0:w532:dbl[])
                    n180 = Rotate 1D Array(1:w527, 2:w518) -> (0:w530:dbl[])
                    n181 = Rotate 1D Array(1:w524, 2:w518) -> (0:w522:dbl[])
                    n182 = Rotate 1D Array(1:w521, 2:w518) -> (0:w520:dbl[])
                    n183 = Replace Array Subset(array=w535, new element=w534, index=w511) -> (w507:timestamp[])
                    n184 = Replace Array Subset(array=w533, new element=w523, index=w511) -> (w517:dbl[])
                    n185 = Replace Array Subset(array=w532, new element=w531, index=w511) -> (w515:dbl[])
                    n186 = Replace Array Subset(array=w530, new element=w529, index=w511) -> (w512:dbl[])
                    n187 = Replace Array Subset(array=w522, new element=w528, index=w511) -> (w505:dbl[])
                    n188 = Replace Array Subset(array=w520, new element=w519, index=w511) -> (w509:dbl[])
                    n189 = Build Cluster Array(w507, w505) -> (→"Depth":T1)
                    n190 = Build Cluster Array(w507, w515) -> (→"Temperature":T1)
                    n191 = Build Cluster Array(w507, w512) -> (→"Conductivity":T1)
                    n192 = Multiply(x=w509, y=750.0) -> (x*y=w508:dbl[])
                    n193 = Build Cluster Array(w507, w508) -> (→"Alti Range":T1)
                  }
                  frame #1 {
                    n194 = Array Size(array=w540) -> (size(s)=w538:i32)
                    n195 = Greater?(x=w538, y=1) -> (0:w537:bool)
                    n196 = case shown="True" w537 {
                      tunnel: w540 -> [_ w557]
                      tunnel: w538 -> [_ w556]
                      tunnel: w539 -> [_ w552]
                      frame False {
                      }
                      frame True {
                        w553 = 0
                        w554 = 1
                        n197 = Subtract(x=w556, y=w554) -> (x-y=w555:i32)
                        n198 = Array Subset(array=w557, index=w554, length=w555) -> (w542:dbl[])
                        n199 = Array Subset(array=w557, index=w553, length=w555) -> (w543:dbl[])
                        n200 = Subtract(x=w543, y=w542) -> (x-y=w546:dbl[])
                        n201 = Array Subset(array=w552, index=w554, length=w555) -> (w548:timestamp[])
                        n202 = Array Subset(array=w552, index=w553, length=w555) -> (w550:timestamp[])
                        n203 = To Double Precision Float(number=w548) -> (double precision float=w547:dbl[])
                        n204 = To Double Precision Float(number=w550) -> (double precision float=w549:dbl[])
                        n205 = Subtract(x=w547, y=w549) -> (x-y=w551:dbl[])
                        n206 = Divide(x=w546, y=w551) -> (x/y=w544:dbl[])
                        n207 = Build Cluster Array(w548, w544) -> (→"Dz/Dt":T1)
                      }
                    }
                  }
                }
                n208 = case shown="True" w495 {
                  tunnel: w492 -> [_ w560]
                  frame False {
                  }
                  frame True {
                    n209 = Get Date/Time In Seconds() -> (seconds since 1Jan1904=→"Time @ max":timestamp)
                    n210 = property on="Payout" class="Slide (strict)"() -> ("Value"=→"Max payout":dbl)  [unwired: 2 in, 2 out]
                    "Max depth" <- w560
                  }
                }
                n211 = case shown="False" w494 {
                  frame False {
                    n212 = property on="Max depth" class="DigNum (strict)"("Value"=0.0) -> ()  [unwired: 2 in, 2 out]
                  }
                  frame True {
                  }
                }
              }
              frame True {
                # "If CTD is emtpy string: increment CTD Miss count, and blink CTD bar"
                n213 = property on="CTD Miss Count" class="DigNum (strict)"() -> ("Value"=w571:dbl)  [unwired: 2 in, 2 out]
                n214 = Increment(x=w571) -> (x+1=w569:dbl)
                n215 = Greater?(x=w569, y=1) -> (0:w561:bool)
                n216 = property on="Depth" class="Slide (strict)"("Blinking"=w561) -> ()  [unwired: 2 in, 2 out]
                n217 = property on="CTD data" class="Str"("Blinking"=w561) -> ()  [unwired: 2 in, 2 out]
                n218 = property on="CTD Miss Count" class="DigNum (strict)"("Value"=w569) -> ()  [unwired: 2 in, 2 out]
                n219 = property on="Depth" class="XYGraph (strict)"("Blinking"=w561) -> ()  [unwired: 2 in, 2 out]
                n220 = property on="Conductivity" class="XYGraph (strict)"("Blinking"=w561) -> ()  [unwired: 2 in, 2 out]
                n221 = property on="Temperature" class="XYGraph (strict)"("Blinking"=w561) -> ()  [unwired: 2 in, 2 out]
                n222 = property on="Dz/Dt" class="XYGraph (strict)"("Blinking"=w561) -> ()  [unwired: 2 in, 2 out]
              }
            }
          }
        }
      }
      frame #7 {
        # "Depth warning system"
        n223 = property on="Drive by \nCTD Data" class="Bool (strict)"() -> ("Value"=w573:bool)  [unwired: 2 in, 2 out]
        n224 = property on="Enabled" class="Bool (strict)"() -> ("Value"=w572:bool)  [unwired: 2 in, 2 out]
        n225 = And(x=w573, y=w572) -> (x .and. y?=w574:bool)
        n226 = case shown="True" w574 {
          selector: w574 -> [w576 _]
          frame False {
            n227 = property on="Alti Range" class="XYGraph (strict)"("Blinking"=w576) -> ()  [unwired: 2 in, 2 out]
            n228 = property on="Too late" class="Str"("Visible"=w576) -> ()  [unwired: 2 in, 2 out]
            n229 = property on="Going up? \ntry to stop at current depth" class="Bool (strict)"("DisabledEnum"=2) -> ()  [unwired: 2 in, 2 out]
          }
          frame True {
            # "Going down"
            n230 = property on="Winch Action Status" class="Enum (strict)"() -> ("Value"=w581:T2)  [unwired: 2 in, 2 out]
            n231 = Equal?(x=w581, y=5) -> (x = y?=w579:bool)
            n232 = Equal?(x=w581, y=4) -> (x = y?=w578:bool)
            n233 = Not(x=w578) -> (.not. x?=w577:bool)
            n234 = global write "isPlaying.vi" "AllBellsShouldStop"(w577) -> ()
            n235 = case shown="True" w578 {
              selector: w578 -> [w589 _]
              frame False {
                n236 = property on="Alti Range" class="XYGraph (strict)"("Blinking"=w589) -> ()  [unwired: 2 in, 2 out]
                n237 = property on="Too late" class="Str"("Visible"=w589) -> ()  [unwired: 2 in, 2 out]
                n238 = global write "isPlaying.vi" "isSoundPlaying"(w589) -> ()
              }
              frame True {
                # "Beep when the altimeter reaches 50m"
                n239 = property on="Current Range" class="DigNum (strict)"() -> ("Value"=w590:dbl)  [unwired: 2 in, 2 out]
                n240 = Less Or Equal?(x=w590, y=35.0) -> (x <= y?=w603:bool)
                n241 = Less Or Equal?(x=w590, y=-5.0) -> (x <= y?=w597:bool)
                n242 = property on="Too late" class="Str"("Visible"=w597) -> ()  [unwired: 2 in, 2 out]
                n243 = Greater Or Equal?(x=w590, y=17.0) -> (x >= y?=w601:bool)
                n244 = And(x=w603, y=w601) -> (x .and. y?=w596:bool)
                n245 = Less Or Equal?(x=w590, y=17.0) -> (x <= y?=w599:bool)
                n246 = case shown="True" w596 {
                  selector: w596 -> [w610 w612]
                  frame False {
                    n247 = Not(x=w610) -> (.not. x?=w611:bool)
                    n248 = global write "isPlaying.vi" "35mBellShouldStop"(w611) -> ()
                  }
                  frame True {
                    n249 = stacked-sequence {
                      tunnel: w612 -> [w613 _]
                      frame #0 {
                        n250 = Not(x=w613) -> (.not. x?=w614:bool)
                        n251 = global write "isPlaying.vi" "50mBellShouldStop"(w613) -> ()
                        n252 = global write "isPlaying.vi" "15mBellShouldStop"(w613) -> ()
                        n253 = global write "isPlaying.vi" "35mBellShouldStop"(w614) -> ()
                      }
                      frame #1 {
                        n254 = call "PlaySoundBelow35m.vi"() -> ()  [unwired: 12 in]
                      }
                    }
                  }
                }
                n255 = case shown="True" w599 {
                  selector: w599 -> [w616 w618]
                  frame False {
                    n256 = Not(x=w616) -> (.not. x?=w617:bool)
                    n257 = property on="Alti Range" class="XYGraph (strict)"("Blinking"=w616) -> ()  [unwired: 2 in, 2 out]
                    n258 = global write "isPlaying.vi" "15mBellShouldStop"(w617) -> ()
                  }
                  frame True {
                    n259 = property on="Alti Range" class="XYGraph (strict)"("Blinking"=w618) -> ()  [unwired: 2 in, 2 out]
                    n260 = stacked-sequence {
                      tunnel: w618 -> [w619 _]
                      frame #0 {
                        n261 = Not(x=w619) -> (.not. x?=w620:bool)
                        n262 = global write "isPlaying.vi" "35mBellShouldStop"(w619) -> ()
                        n263 = global write "isPlaying.vi" "50mBellShouldStop"(w619) -> ()
                        n264 = global write "isPlaying.vi" "15mBellShouldStop"(w620) -> ()
                      }
                      frame #1 {
                        n265 = call "PlaySoundBelow15m.vi"() -> ()  [unwired: 12 in]
                      }
                    }
                  }
                }
                n266 = case shown="True" w597 {
                  frame False {
                  }
                  frame True {
                    "Too late" <- "Too late now!!! Just pray for the best!"
                  }
                }
                n267 = Less Or Equal?(x=w590, y=50.0) -> (x <= y?=w594:bool)
                n268 = Greater Or Equal?(x=w590, y=35.0) -> (x >= y?=w592:bool)
                n269 = And(x=w594, y=w592) -> (x .and. y?=w591:bool)
                n270 = case shown="True" w591 {
                  selector: w591 -> [w605 w607]
                  frame False {
                    n271 = Not(x=w605) -> (.not. x?=w606:bool)
                    n272 = global write "isPlaying.vi" "50mBellShouldStop"(w606) -> ()
                  }
                  frame True {
                    n273 = stacked-sequence {
                      tunnel: w607 -> [w608 _]
                      frame #0 {
                        n274 = Not(x=w608) -> (.not. x?=w609:bool)
                        n275 = global write "isPlaying.vi" "35mBellShouldStop"(w608) -> ()
                        n276 = global write "isPlaying.vi" "15mBellShouldStop"(w608) -> ()
                        n277 = global write "isPlaying.vi" "50mBellShouldStop"(w609) -> ()
                      }
                      frame #1 {
                        n278 = call "PlaySoundBelow50m.vi"() -> ()  [unwired: 12 in]
                      }
                    }
                  }
                }
              }
            }
            n279 = case shown="True" w579 {
              frame False {
                n280 = property on="Going up? \ntry to stop at current depth" class="Bool (strict)"("DisabledEnum"=2) -> ()  [unwired: 2 in, 2 out]
              }
              frame True {
                # "Going up"
                n281 = property on="Going up? \ntry to stop at current depth" class="Bool (strict)"("DisabledEnum"=0) -> ()  [unwired: 2 in, 2 out]
                n282 = case shown="True" "Going up? \ntry to stop at current depth" {
                  frame False {
                  }
                  frame True {
                    n283 = property on="Payout" class="Slide (strict)"() -> ("Value"=w588:dbl)  [unwired: 2 in, 2 out]
                    n284 = Subtract(x=w588, y=10.0) -> (x-y=w587:dbl)
                    n285 = property on="Min. payout [turns]" class="DigNum (strict)"("Val(Sgnl)"=w587) -> ()  [unwired: 2 in, 2 out]
                  }
                }
              }
            }
          }
        }
      }
      frame #8 {
        # "Check for dead com links"
        n286 = stacked-sequence {
          seq-local: [w627 _] -> [_ w644]
          tunnel: w625 -> [w628 _]
          tunnel: [_ w644] -> w624
          tunnel: w623 -> [_ w645]
          tunnel: [_ w643] -> w622
          tunnel: w621 -> [w626 _]
          frame #0 {
            # "If winch miss count > 25, close connection and open again"
            n287 = property on="Winch Miss Count" class="DigNum (strict)"() -> ("Value"=w631:dbl)  [unwired: 2 in, 2 out]
            n288 = Greater?(x=w631, y=25) -> (0:w629:bool)
            n289 = case shown="True" w629 {
              tunnel: w628 -> [w632 w635]
              tunnel: [w632 w634] -> w627
              tunnel: w626 -> [_ w633]
              frame False {
              }
              frame True {
                n290 = stacked-sequence {
                  tunnel: w635 -> [w637 _ _]
                  tunnel: [_ _ w640] -> w634
                  tunnel: w633 -> [_ _ w638]
                  frame #0 {
                    n291 = TCP Close Connection(connection ID=w637) -> (error out=w636:errorcluster)  [unwired: 2 in, 1 out]
                    n292 = call <vilib>:"Clear Errors.vi"("error in (no error)"=w636) -> ()  [unwired: 5 in, 2 out]
                  }
                  frame #1 {
                    n293 = call "Time Delay"() -> ()  [unwired: 11 in, 1 out]
                  }
                  frame #2 {
                    n294 = TCP Open Connection(address=w638, remote port or service name=4050, timeout ms (60000)=1000) -> (connection ID=w640:refnum<k5>, error out=w639:errorcluster)  [unwired: 2 in]
                    n295 = call <vilib>:"Clear Errors.vi"("error in (no error)"=w639) -> ()  [unwired: 5 in, 2 out]
                  }
                }
              }
            }
          }
          frame #1 {
            # "If CTD miss count > 10, close connection and open again"
            n296 = property on="CTD Miss Count" class="DigNum (strict)"() -> ("Value"=w646:dbl)  [unwired: 2 in, 2 out]
            n297 = Greater?(x=w646, y=10) -> (0:w648:bool)
            n298 = case shown="True" w648 {
              tunnel: w645 -> [w649 w651]
              tunnel: [w649 w650] -> w643
              frame False {
              }
              frame True {
                n299 = stacked-sequence {
                  tunnel: w651 -> [w653 _ _ _]
                  tunnel: [_ _ _ w658] -> w650
                  frame #0 {
                    n300 = TCP Close Connection(connection ID=w653) -> (error out=w652:errorcluster)  [unwired: 2 in, 1 out]
                    n301 = call <vilib>:"Clear Errors.vi"("error in (no error)"=w652) -> ()  [unwired: 5 in, 2 out]
                  }
                  frame #1 {
                    n302 = call "Time Delay2"() -> ()  [unwired: 11 in, 1 out]
                  }
                  frame #2 {
                    n303 = property on="CTD Miss Count" class="DigNum (strict)"("Value"=0) -> ()  [unwired: 2 in, 2 out]
                  }
                  frame #3 {
                    n304 = property on="Port" class="DigNum (strict)"() -> ("Value"=w656:i32)  [unwired: 2 in, 2 out]
                    n305 = property on="CTD Data  IP Address" class="Str"() -> ("Value"=w657:string)  [unwired: 2 in, 2 out]
                    n306 = TCP Open Connection(address=w657, remote port or service name=w656, timeout ms (60000)=1000) -> (connection ID=w658:refnum<k5>, error out=w655:errorcluster)  [unwired: 2 in]
                    n307 = call <vilib>:"Clear Errors.vi"("error in (no error)"=w655) -> ()  [unwired: 5 in, 2 out]
                  }
                }
              }
            }
          }
        }
      }
      frame #9 {
        # "Check if the values set by the user \nand the values on the controls are the same"
        # "Image Capture of the Front Panel"
        n308 = property on="Enabled" class="Bool (strict)"() -> ("Value"=w664:bool)  [unwired: 2 in, 2 out]
        n309 = case shown="True" w664 {
          frame False {
          }
          frame True {
            n310 = property on="Min payout" class="DigNum (strict)"() -> ("Value"=w718:dbl)  [unwired: 2 in, 2 out]
            n311 = property on="Min. payout [turns]" class="DigNum (strict)"() -> ("Value"=w717:dbl)  [unwired: 2 in, 2 out]
            n312 = property on="Wire in speed" class="DigNum (strict)"() -> ("Value"=w710:dbl)  [unwired: 2 in, 2 out]
            n313 = property on="Wire in speed\n[turns/sec]" class="DigNum (strict)"() -> ("Value"=w709:dbl)  [unwired: 2 in, 2 out]
            n314 = property on="Max. payout [turns]" class="DigNum (strict)"() -> ("Value"=w716:dbl)  [unwired: 2 in, 2 out]
            n315 = property on="Max payout" class="DigNum (strict)"() -> ("Value"=w715:dbl)  [unwired: 2 in, 2 out]
            n316 = property on="Vel out Init. [turns/sec]" class="DigNum (strict)"() -> ("Value"=w713:dbl)  [unwired: 2 in, 2 out]
            n317 = property on="Wire out speed" class="DigNum (strict)"() -> ("Value"=w712:dbl)  [unwired: 2 in, 2 out]
            n318 = Not Equal?(x=w717, y=w718) -> (x != y?=w719:bool)
            n319 = Not Equal?(x=w710, y=w709) -> (x != y?=w708:bool)
            n320 = Not Equal?(x=w716, y=w715) -> (x != y?=w714:bool)
            n321 = Not Equal?(x=w713, y=w712) -> (x != y?=w711:bool)
            n322 = property on="Min. payout [turns]" class="DigNum (strict)"("Blinking"=w719) -> ()  [unwired: 2 in, 2 out]
            n323 = property on="Min payout" class="DigNum (strict)"("Blinking"=w719) -> ()  [unwired: 2 in, 2 out]
            n324 = property on="Wire in speed\n[turns/sec]" class="DigNum (strict)"("Blinking"=w708) -> ()  [unwired: 2 in, 2 out]
            n325 = property on="Max. payout [turns]" class="DigNum (strict)"("Blinking"=w714) -> ()  [unwired: 2 in, 2 out]
            n326 = property on="Vel out Init. [turns/sec]" class="DigNum (strict)"("Blinking"=w711) -> ()  [unwired: 2 in, 2 out]
            n327 = property on="Wire in speed" class="DigNum (strict)"("Blinking"=w708) -> ()  [unwired: 2 in, 2 out]
            n328 = property on="Max payout" class="DigNum (strict)"("Blinking"=w714) -> ()  [unwired: 2 in, 2 out]
            n329 = property on="Wire out speed" class="DigNum (strict)"("Blinking"=w711) -> ()  [unwired: 2 in, 2 out]
            n330 = property on="Stop decel out" class="DigNum (strict)"() -> ("Value"=w686:dbl)  [unwired: 2 in, 2 out]
            n331 = property on="Decel stop out" class="DigNum (strict)"() -> ("Value"=w685:dbl)  [unwired: 2 in, 2 out]
            n332 = property on="Final in speed" class="DigNum (strict)"() -> ("Value"=w707:dbl)  [unwired: 2 in, 2 out]
            n333 = property on="Final in speed\n[turns/sec]" class="DigNum (strict)"() -> ("Value"=w706:dbl)  [unwired: 2 in, 2 out]
            n334 = property on="Accel in" class="DigNum (strict)"() -> ("Value"=w701:dbl)  [unwired: 2 in, 2 out]
            n335 = property on="Accel  in" class="DigNum (strict)"() -> ("Value"=w700:dbl)  [unwired: 2 in, 2 out]
            n336 = property on="Accel out" class="DigNum (strict)"() -> ("Value"=w698:dbl)  [unwired: 2 in, 2 out]
            n337 = property on="Accel out" class="DigNum (strict)"() -> ("Value"=w697:dbl)  [unwired: 2 in, 2 out]
            n338 = Not Equal?(x=w686, y=w685) -> (x != y?=w684:bool)
            n339 = Not Equal?(x=w707, y=w706) -> (x != y?=w705:bool)
            n340 = Not Equal?(x=w701, y=w700) -> (x != y?=w699:bool)
            n341 = Not Equal?(x=w698, y=w697) -> (x != y?=w696:bool)
            n342 = property on="Stop decel out" class="DigNum (strict)"("Blinking"=w684) -> ()  [unwired: 2 in, 2 out]
            n343 = property on="Decel stop out" class="DigNum (strict)"("Blinking"=w684) -> ()  [unwired: 2 in, 2 out]
            n344 = property on="Final in speed" class="DigNum (strict)"("Blinking"=w705) -> ()  [unwired: 2 in, 2 out]
            n345 = property on="Final in speed\n[turns/sec]" class="DigNum (strict)"("Blinking"=w705) -> ()  [unwired: 2 in, 2 out]
            n346 = property on="Accel  in" class="DigNum (strict)"("Blinking"=w699) -> ()  [unwired: 2 in, 2 out]
            n347 = property on="Accel out" class="DigNum (strict)"("Blinking"=w696) -> ()  [unwired: 2 in, 2 out]
            n348 = property on="Accel in" class="DigNum (strict)"("Blinking"=w699) -> ()  [unwired: 2 in, 2 out]
            n349 = property on="Accel out" class="DigNum (strict)"("Blinking"=w696) -> ()  [unwired: 2 in, 2 out]
            n350 = property on="Decel stop in" class="DigNum (strict)"() -> ("Value"=w689:dbl)  [unwired: 2 in, 2 out]
            n351 = property on="Stop decel in" class="DigNum (strict)"() -> ("Value"=w688:dbl)  [unwired: 2 in, 2 out]
            n352 = property on="Decel in" class="DigNum (strict)"() -> ("Value"=w695:dbl)  [unwired: 2 in, 2 out]
            n353 = property on="Decel in" class="DigNum (strict)"() -> ("Value"=w694:dbl)  [unwired: 2 in, 2 out]
            n354 = property on="Decel out" class="DigNum (strict)"() -> ("Value"=w692:dbl)  [unwired: 2 in, 2 out]
            n355 = property on="Decel out" class="DigNum (strict)"() -> ("Value"=w691:dbl)  [unwired: 2 in, 2 out]
            n356 = property on="Slow payout (up)" class="DigNum (strict)"() -> ("Value"=w704:dbl)  [unwired: 2 in, 2 out]
            n357 = property on="Slow payout (up)\n[turns]" class="DigNum (strict)"() -> ("Value"=w703:dbl)  [unwired: 2 in, 2 out]
            n358 = Not Equal?(x=w689, y=w688) -> (x != y?=w687:bool)
            n359 = Not Equal?(x=w695, y=w694) -> (x != y?=w693:bool)
            n360 = Not Equal?(x=w692, y=w691) -> (x != y?=w690:bool)
            n361 = Not Equal?(x=w704, y=w703) -> (x != y?=w702:bool)
            n362 = property on="Stop decel in" class="DigNum (strict)"("Blinking"=w687) -> ()  [unwired: 2 in, 2 out]
            n363 = property on="Decel in" class="DigNum (strict)"("Blinking"=w693) -> ()  [unwired: 2 in, 2 out]
            n364 = property on="Decel out" class="DigNum (strict)"("Blinking"=w690) -> ()  [unwired: 2 in, 2 out]
            n365 = property on="Decel stop in" class="DigNum (strict)"("Blinking"=w687) -> ()  [unwired: 2 in, 2 out]
            n366 = property on="Decel in" class="DigNum (strict)"("Blinking"=w693) -> ()  [unwired: 2 in, 2 out]
            n367 = property on="Decel out" class="DigNum (strict)"("Blinking"=w690) -> ()  [unwired: 2 in, 2 out]
            n368 = property on="Slow payout (up)\n[turns]" class="DigNum (strict)"("Blinking"=w702) -> ()  [unwired: 2 in, 2 out]
            n369 = property on="Slow payout (up)" class="DigNum (strict)"("Blinking"=w702) -> ()  [unwired: 2 in, 2 out]
          }
        }
        n370 = Get Date/Time In Seconds() -> (seconds since 1Jan1904=w669:timestamp)
        n371 = Format Date/Time String(seconds (now)=w669) -> (date/time string=w668:string)  [unwired: 2 in]
        n372 = Concatenate Strings("Updated: ", w668) -> (→"Last update string":string)
        n373 = case shown="True" "Screen Capture" {
          frame False {
          }
          frame True {
            n374 = feedback #1() -> (w720:errorcluster)  [unwired: 1 in]
            n375 = call <vilib>:"Check if File or Folder Exists.vi"("error in (no error)"=w720, "path"="Path of Image Capture") -> ("error out"=w722:errorcluster, "file or folder exists?"=w724:bool, "dup path"=w725:path)  [unwired: 7 in]
            n376 = case shown="True" w724 {
              tunnel: w725 -> [w732 w734]
              tunnel: w722 -> [w727 _]
              tunnel: [w726 w733] -> w721
              frame False {
                n377 = Open/Create/Replace File(file path (use dialog)=w732, error in=w727, operation (0:open)=4, access (0:read/write)=0) -> (refnum out=w728:refnum<file>, error out=w729:errorcluster)  [unwired: 2 in, 1 out]
                n378 = Close File(refnum=w728, error in=w729) -> (error out=w726:errorcluster)  [unwired: 1 out]
              }
              frame True {
                # "Close VI ref"
                # "24 bit image depth"
                # "Open VI Reference Function"
                # "Current VI's Path"
                # "Save an image capture of the Fron Panel"
                n379 = Current VI's Path() -> (path=w741:path)
                n380 = Open VI Reference(vi path=w741) -> (vi reference=w738:refnum<vi>, error out=w740:errorcluster)  [unwired: 5 in]
                n381 = invoke class="VI" method="FP.Get Image"(reference=w738, error in=w740, "image depth"=24) -> (reference out=w736:refnum<vi>, error out=w737:errorcluster, "image data"=w739:T5)  [unwired: 3 in, 3 out]
                n382 = Close Reference(reference=w736) -> ()  [unwired: 1 in, 1 out]
                n383 = call <vilib>:"Write PNG File.vi"("error in (no error)"=w737, "image data"=w739, "path to PNG file"=w734) -> ("error out"=w733:errorcluster)  [unwired: 7 in, 1 out]
              }
            }
            n384 = feedback-in #1(w721) -> ()
          }
        }
        n385 = stacked-sequence {
          tunnel: w660 -> [_ w680]
          tunnel: w661 -> [w671 w682]
          tunnel: w663 -> [w672 _]
          tunnel: w662 -> [_ _]
          frame #0 {
            n386 = Build Cluster Array(w671, w672) -> (→"Payout History":T1)
          }
          frame #1 {
            n387 = To Double Precision Float(number=w682) -> (double precision float=w681:dbl[])
            n388 = To Double Precision Float(number=w680) -> (double precision float=w679:dbl[])
            n389 = Build Array(w681, w679) -> (w683:dbl[][])
            n390 = Array Max & Min(array=w683) -> (max value=w678:dbl, min value=w674:dbl)  [unwired: 2 out]
            n391 = property on="Dz/Dt" class="XYGraph (strict)"("XScale.Minimum"=w674) -> ()  [unwired: 2 in, 2 out]
            n392 = property on="Depth" class="XYGraph (strict)"("XScale.Minimum"=w674) -> ()  [unwired: 2 in, 2 out]
            n393 = property on="Conductivity" class="XYGraph (strict)"("XScale.Minimum"=w674) -> ()  [unwired: 2 in, 2 out]
            n394 = property on="Temperature" class="XYGraph (strict)"("XScale.Minimum"=w674) -> ()  [unwired: 2 in, 2 out]
            n395 = property on="Payout History" class="XYGraph (strict)"("XScale.Minimum"=w674) -> ()  [unwired: 2 in, 2 out]
            n396 = Subtract(x=w678, y=w674) -> (x-y=w677:dbl)
            n397 = Divide(x=w677, y=2.0) -> (x/y=w675:dbl)
            n398 = Add(x=w675, y=w674) -> (x+y=w673:dbl)
            n399 = property on="Depth" class="XYGraph (strict)"("XScale.Maximum"=w678) -> ()  [unwired: 2 in, 2 out]
            n400 = property on="Payout History" class="XYGraph (strict)"("XScale.Maximum"=w678) -> ()  [unwired: 2 in, 2 out]
            n401 = property on="Temperature" class="XYGraph (strict)"("XScale.Maximum"=w678) -> ()  [unwired: 2 in, 2 out]
            n402 = property on="Alti Range" class="XYGraph (strict)"("XScale.Maximum"=w678) -> ()  [unwired: 2 in, 2 out]
            n403 = property on="Conductivity" class="XYGraph (strict)"("XScale.Maximum"=w678) -> ()  [unwired: 2 in, 2 out]
            n404 = property on="Dz/Dt" class="XYGraph (strict)"("XScale.Maximum"=w678) -> ()  [unwired: 2 in, 2 out]
            n405 = property on="Alti Range" class="XYGraph (strict)"("XScale.Minimum"=w673) -> ()  [unwired: 2 in, 2 out]
          }
        }
      }
    }
  }
  n406 = Strip Path(path=w15) -> (stripped path=w14:path)  [unwired: 1 out]
  n407 = Build Path(base path=w14, name or relative path="Sites") -> (appended path=w12:path)
  n408 = Build Path(base path=w12, name or relative path="FCTD_WINCH") -> (appended path=w10:path)
  n409 = Build Path(base path=w10, name or relative path="LabView.png") -> (appended path=w8:path)
  n410 = property on="Path of Image Capture" class="Path"("Value"=w8) -> ()  [unwired: 2 in, 2 out]
  n411 = TCP Close Connection(connection ID=w24, error in (no error)=w57) -> (error out=w26:errorcluster)  [unwired: 1 in, 1 out]
  n412 = TCP Close Connection(connection ID=w33, error in (no error)=w31) -> (error out=w35:errorcluster)  [unwired: 1 in, 1 out]
  n413 = call <vilib>:"Simple Error Handler.vi"("error in (no error)"=w26) -> ()  [unwired: 4 in, 5 out]
  n414 = call <vilib>:"Simple Error Handler.vi"("error in (no error)"=w35) -> ()  [unwired: 4 in, 5 out]
  "CTD Miss Count" <- w25
  "Winch Miss Count" <- w25
  "RL Status Received" <- FALSE
